vi "EnFlo_Tunnel_Display.vi"(4 "End Time":dbl, 5 "Start Time":dbl, 6 "Channel Values":dbl[](array[numeric]) format="%.3f", 7 "Ch names":string[](array[string])) -> ()   [LabVIEW 2015]
uses:
  Anemometry Sub Vis/Data_plotting_vis/File_Template_Clus.ctl
  Anemometry Sub Vis/Controls/Global_mode.ctl
  Anemometry Sub Vis/Globals/Constants_global.vi
  Anemometry Sub Vis/Data_plotting_vis/Results_plotter_Global.vi
  <vilib>/gmath/NI_Gmath.lvlib
panel:
  out "Averaging time (minutes)":dbl format="%#.1f"
  out "End time":timestamp format="%<%H:%M\n%x>T"
  out "Start time":timestamp format="%<%H:%M\n%x>T"
  out "Top Level":bool
  out "Loop number":i32
  out "Lateral profiles":cluster{"Y Axis Current":dbl[], dbl[]}[](graph)
  out "Setpoints":dbl[](array[numeric])
  in  "Subtract Setpoint?":bool
  out "Vert Disp (mm)  @ 14m":dbl
  out "Inlet St Dev":dbl format="%#.3g"
  out "Inlet mapping":dbl[][](graph)=[[0.00729, 0.18153463174730816, 0.17352738437348433, 1.6752433719500537, 8.231465735195274, 17.570357598383207, 23.099772817121426, 25.58386930448374, 25.31727725753219, 24.28926231541072, 18.717383219374323, 10.355253339797807, 2.7760273383248344, 0.3109897541921306, 0.08276881403435009, 0.06197], [0.04411, 0.1361526368018142, 0.04039202183336771, 1.5611636795339547, 8.176972694107874, 17.32000974741714, 24.257541358764026, 25.949153465972987, 26.01802540761648, 25.060373307424115, 18.284750328365213, 8.689831176707928, 2.642937641487066, 0.43219350072447926, -0.019957690739617468, 0.07351], [0.05478, 0.03446320268089581, 0.2086595806581808, 1.6919212249796047, 6.580368005180591, 14.333585185483123, 21.06810094963999, 23.709254571137723, 24.04768940379576, 21.01660820522005, 13.60443428327954, 6.2766496258038735, 1.7988963349022484, 0.2952877651784204, 0.05436788410934033, 0.1022], [0.04013, 0.06419557464541133, 0.2035068586120256, 1.3118741659450193, 4.7061387064566835, 9.009825946069038, 12.927700276268434, 17.003135081884164, 16.83885730812343, 12.902263313363814, 8.246161922417906, 4.035269404379355, 1.329605659745338, 0.24574055091433544, 0.012829784119986217, 0.08755], [0.04404, 0.022691144295571734, 0.19102098261858932, 0.8525411026079828, 2.2353542219792946, 3.966676465246214, 6.305347763088489, 8.17672908183636, 7.7348668140659, 5.703994479070454, 3.8329088824353237, 1.9256956625267279, 0.6611488869641811, 0.20508248283573002, 0.10119553469307395, 0.08441]]
  out "Upstream Floor":cluster{"Array":dbl[], dbl[]}[](graph)
  in  "Averaging time (mins)":dbl=0.5 format="%.2f"
  in  "History in Minutes":dbl
  out "Strat":cluster{dbl[], dbl[]}[](graph)
  out "Des Air Temp":dbl format="%#.2g"
  out "Heat Extraction kW":dbl format="%#.2g"
  out "Av Pre Inlet Temp":dbl format="%#.2g"
  out "Av Exit  Temp":dbl format="%#.2g"
  out "Exit Dem Temp":dbl format="%#.2g"
  out "Heat Exchanger Valve %":dbl format="%#.1f"
  out "Delta T":dbl format="%#.2g"
  out "Pump Speed %":dbl format="%#.0f"
  out "Meas Delta P":dbl format="%#.2g"
  out "Desired Delta P":dbl format="%#.2f"
  out "Return Pressure":dbl format="%#.2g"
  out "Supply Pressure":dbl format="%#.2g"
  out "Max Motor Temp":dbl format="%#.1g"
  out "% Speed Tweak":dbl format="%#.2g"
  out "Shaft RPM":dbl format="%#.2g"
  out "K Factor":dbl format="%#.2g"
  out "Tunnel Speed  m/s":dbl format="%.3g"
  out "Uni Chilled water Temp":dbl format="%#.2g"
  out "Mixing Valve %":dbl format="%#.1f"
  out "Dem Temp":dbl
  out "Return Temp":dbl format="%#.2g"
  out "Supply Temp":dbl format="%#.2g"
  out "Floor_Cooling:Enable":bool
  out "Chiller_Pump:Enable":bool
  out "Panel Temps":cluster{"Array":dbl[], dbl[]}[](graph)
  in  "Stop Button":bool
  out "Heaters Enabled":bool
  out "Inlet Heaters":cluster{"yi":dbl[], dbl[]}[](graph)
  # "Chiller Pump Information"
  # "Chilled Water"
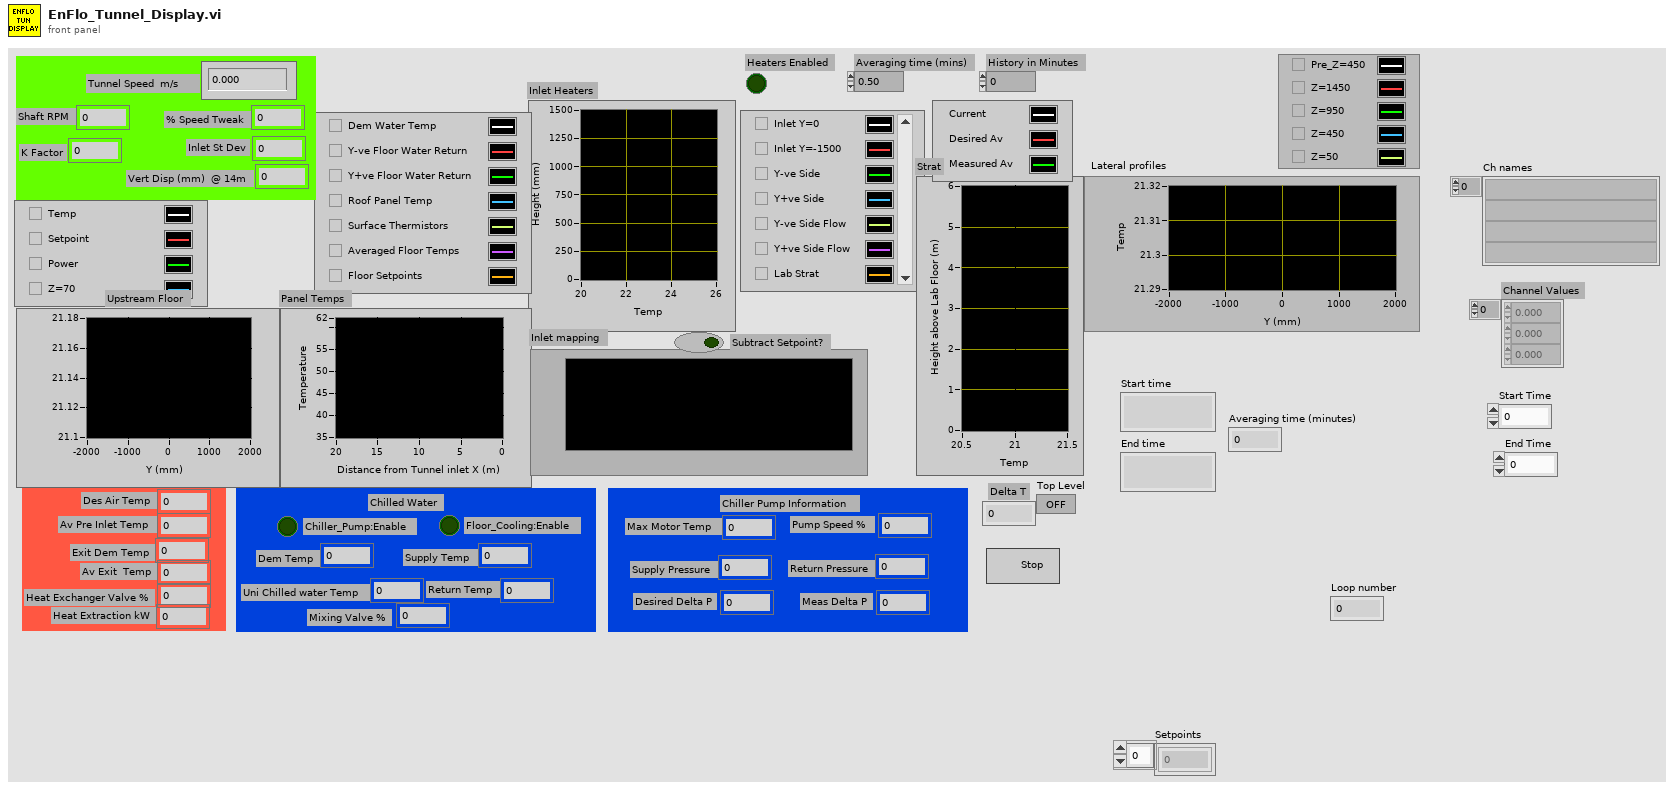
[diagram p1: front panel]
types:
  T1 = typedef "Global_mode.ctl" = enum16{"Read Global", "Load Global From File", "Write Global to File"}
  T2 = typedef "File_Template_Clus.ctl" = cluster{"Template Channel Name":string, "Description":string, "Tolerance":dbl, "Precision":string, "Folder level":string, "Source":string[], "Replace":string[], "Summarise":bool, "Dispose":bool, "Minimum Value":string, "Maths":string, "Omit Rows Containing":string[], "Ignore When":string[]}
  T3 = cluster{"X Max":dbl, "Y Max ":dbl, "X Scale":cluster{"Xo":dbl, "delta X":dbl}, "Y Scale":cluster{"Xo":dbl, "delta X":dbl}, "X Values":dbl[], "Y Values":dbl[], "Z Max":dbl, "Z Min":dbl}
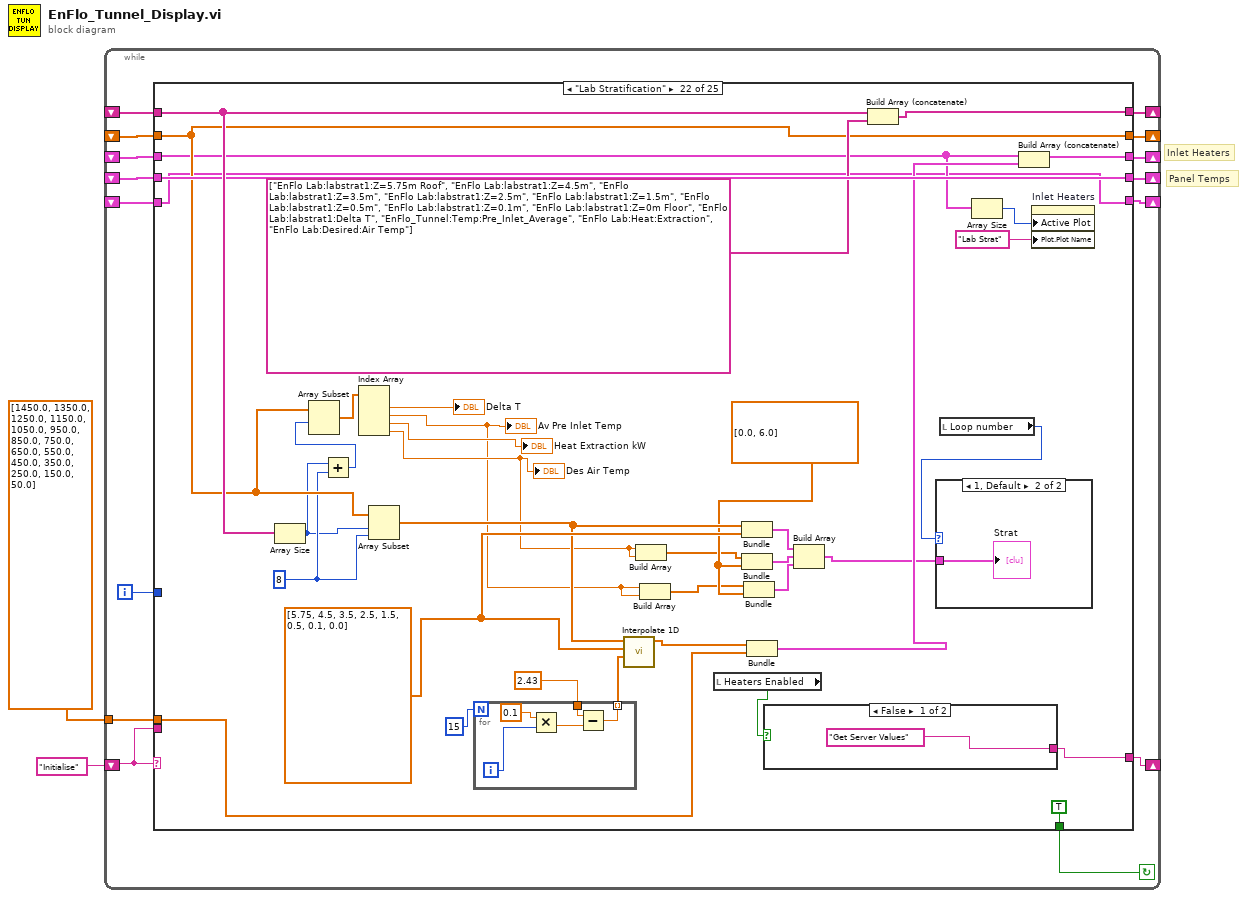
[diagram p0: block diagram]
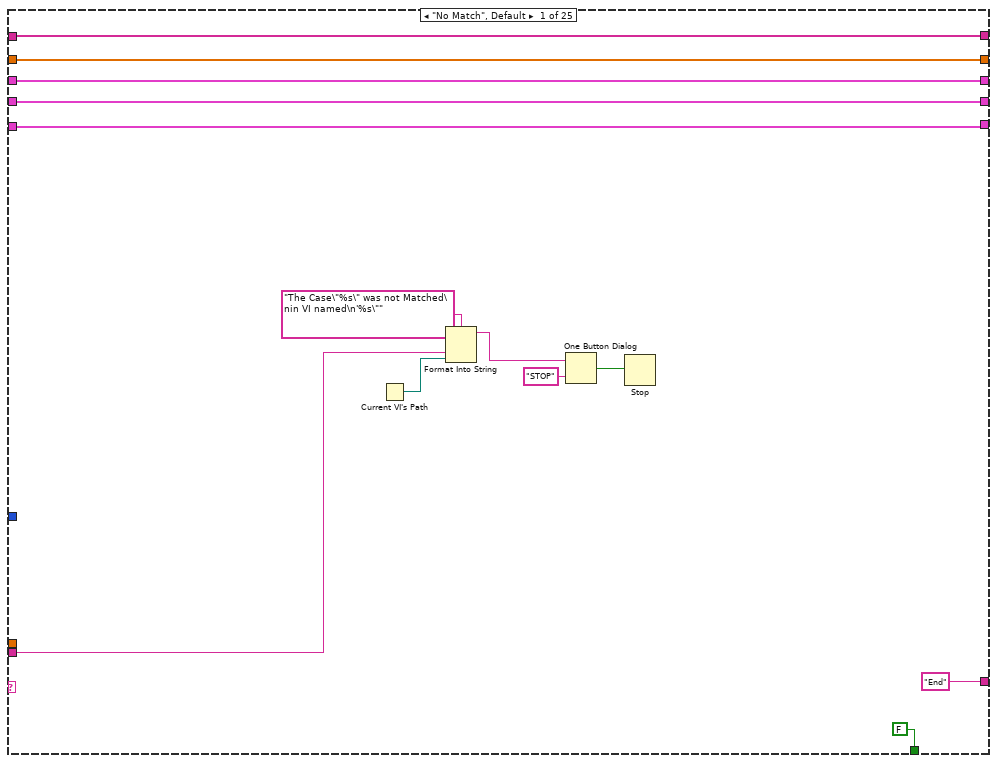
[diagram p2: hidden frame]
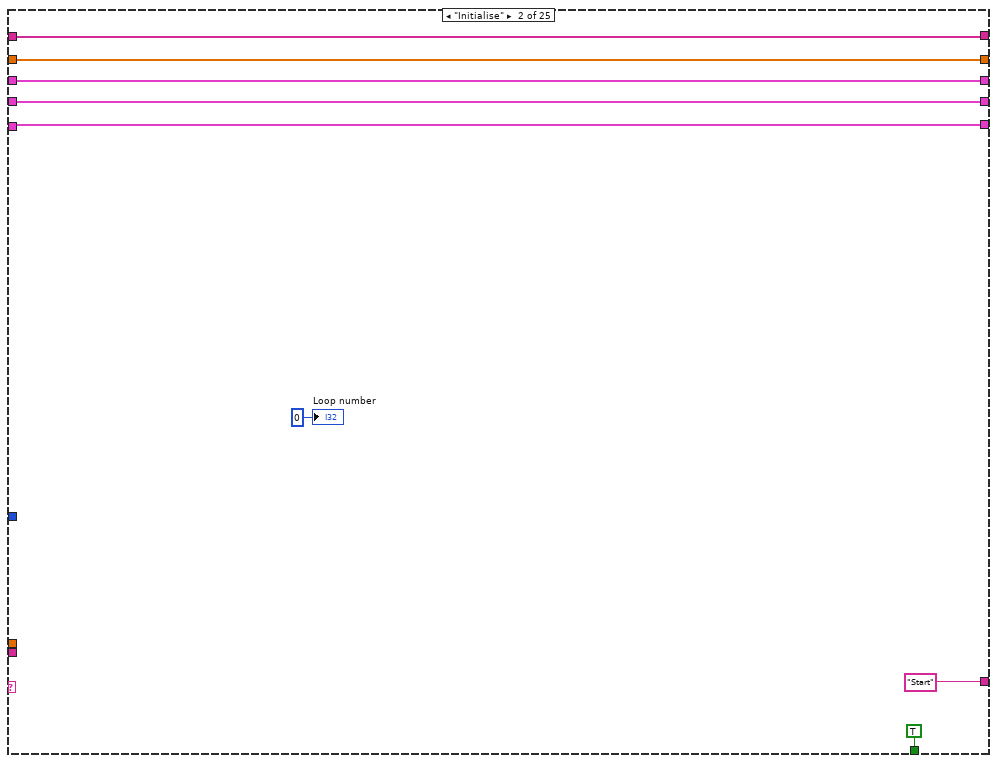
[diagram p3: hidden frame]
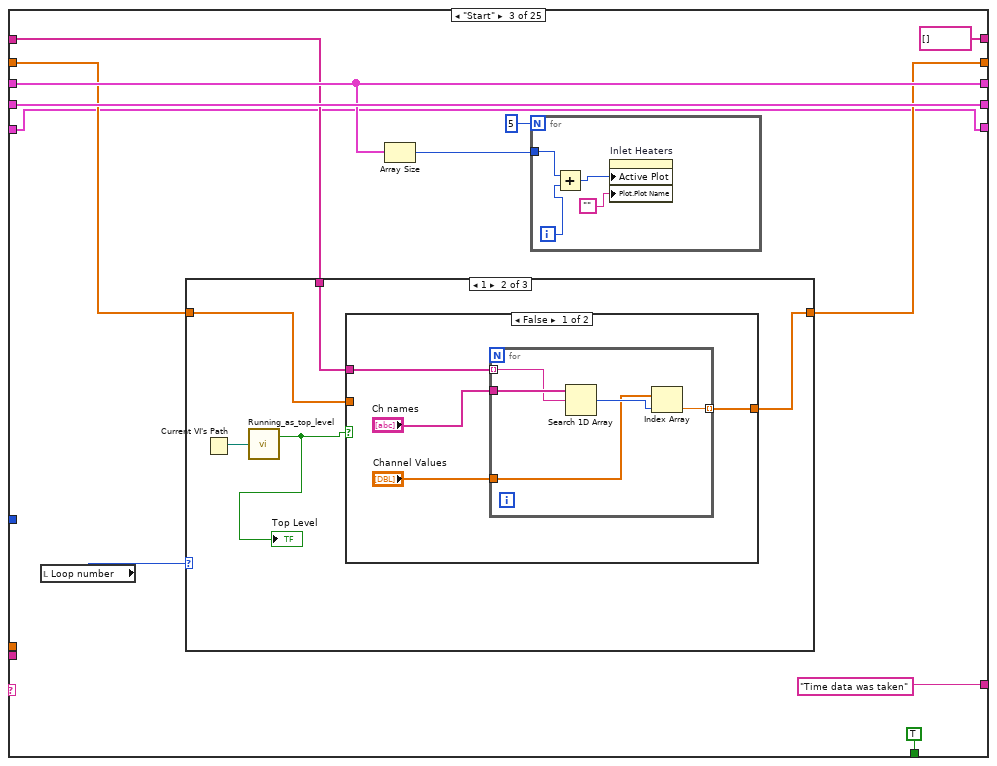
[diagram p4: hidden frame]
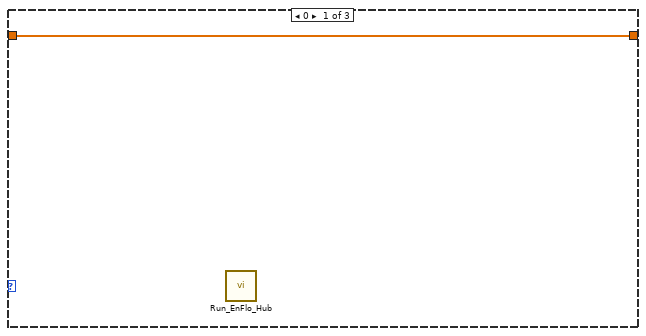
[diagram p5: hidden frame]
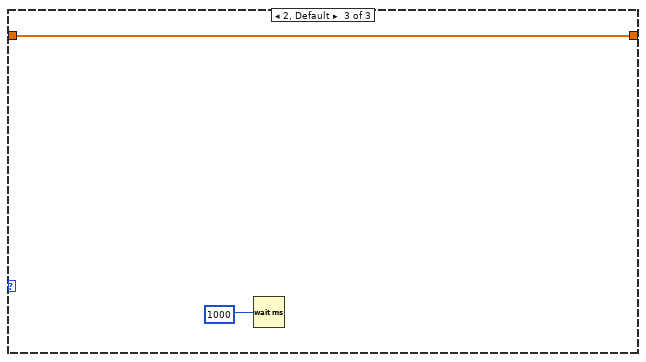
[diagram p7: hidden frame]
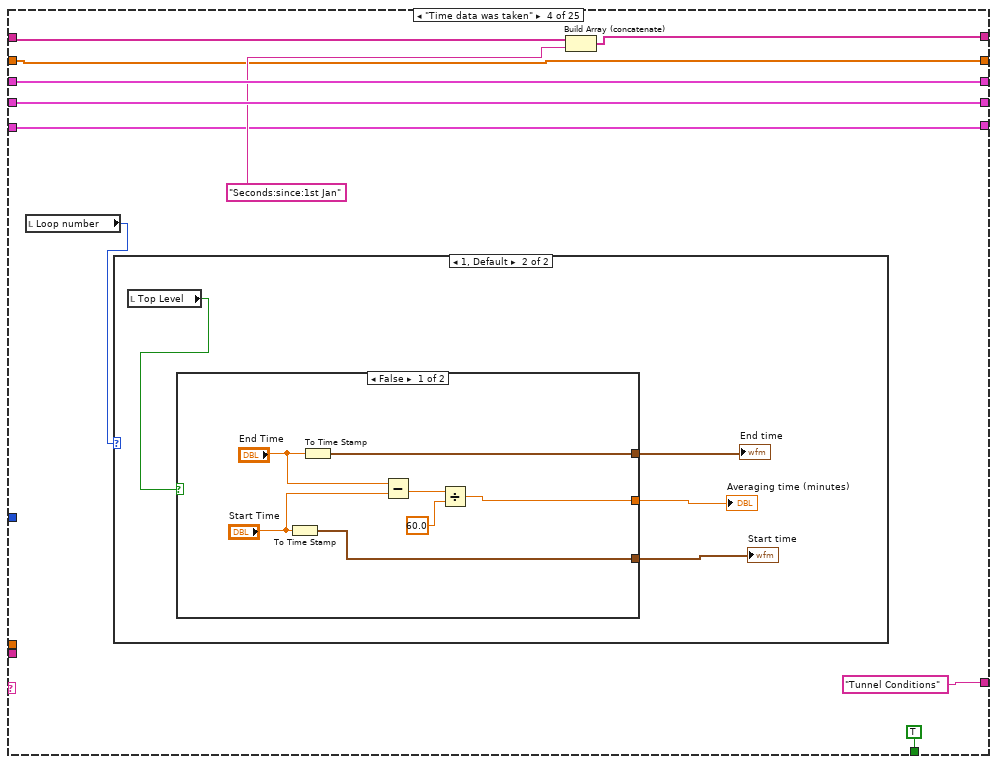
[diagram p8: hidden frame]
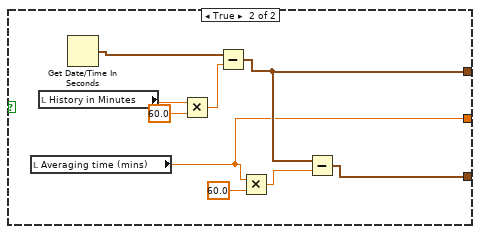
[diagram p10: hidden frame]
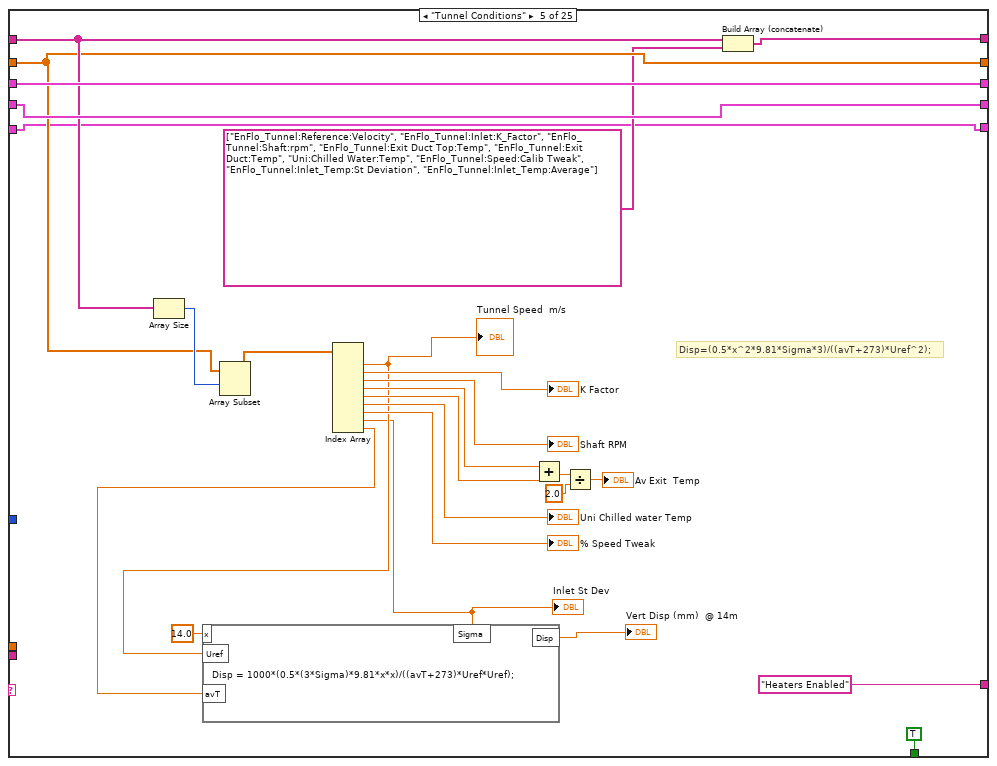
[diagram p11: hidden frame]
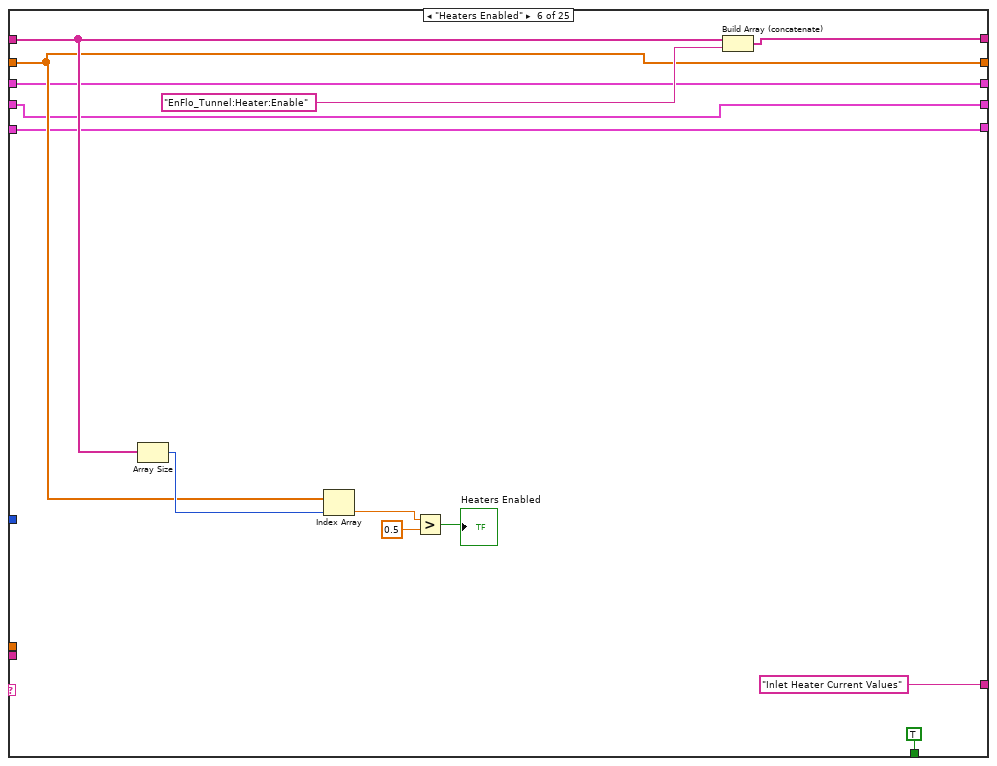
[diagram p12: hidden frame]
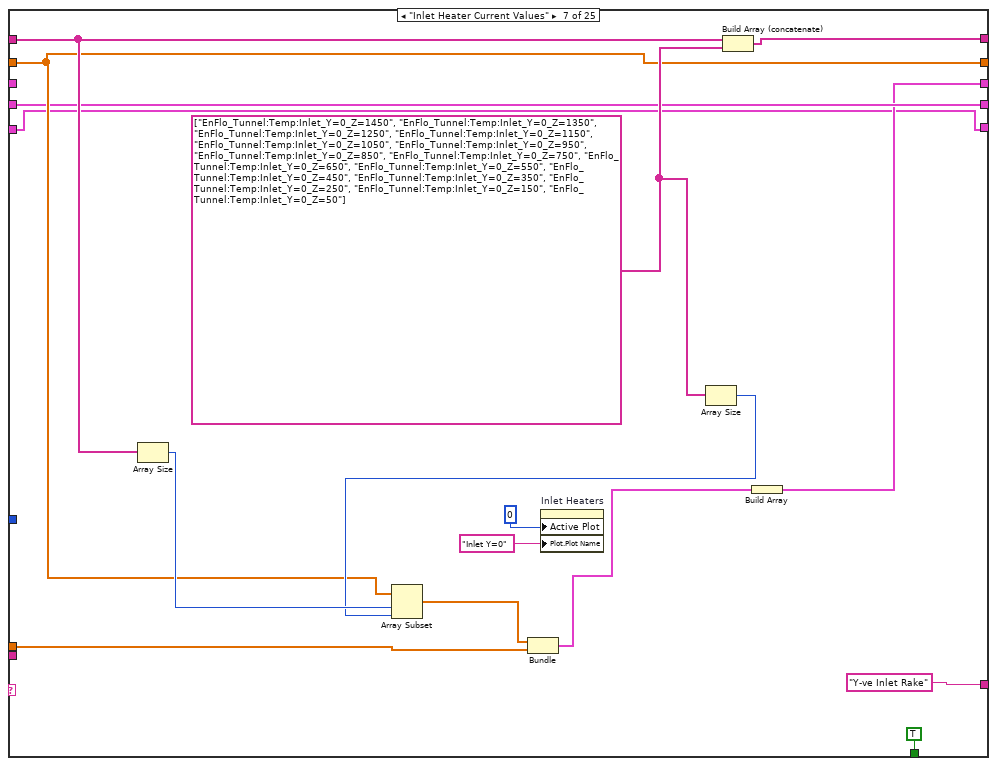
[diagram p13: hidden frame]
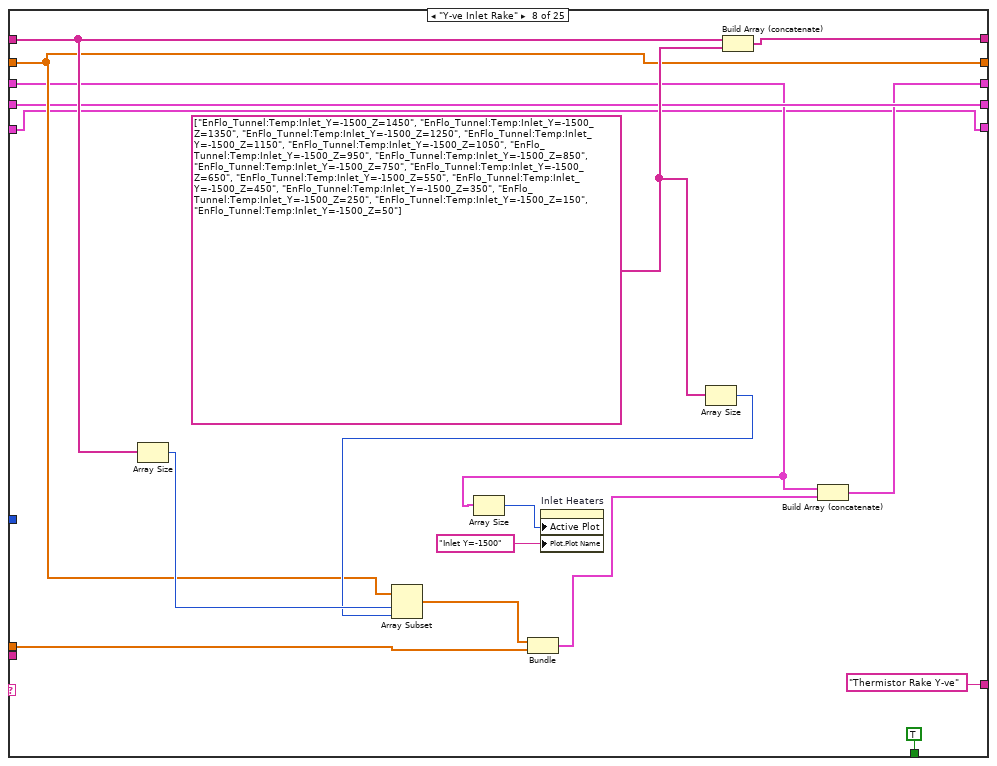
[diagram p14: hidden frame]
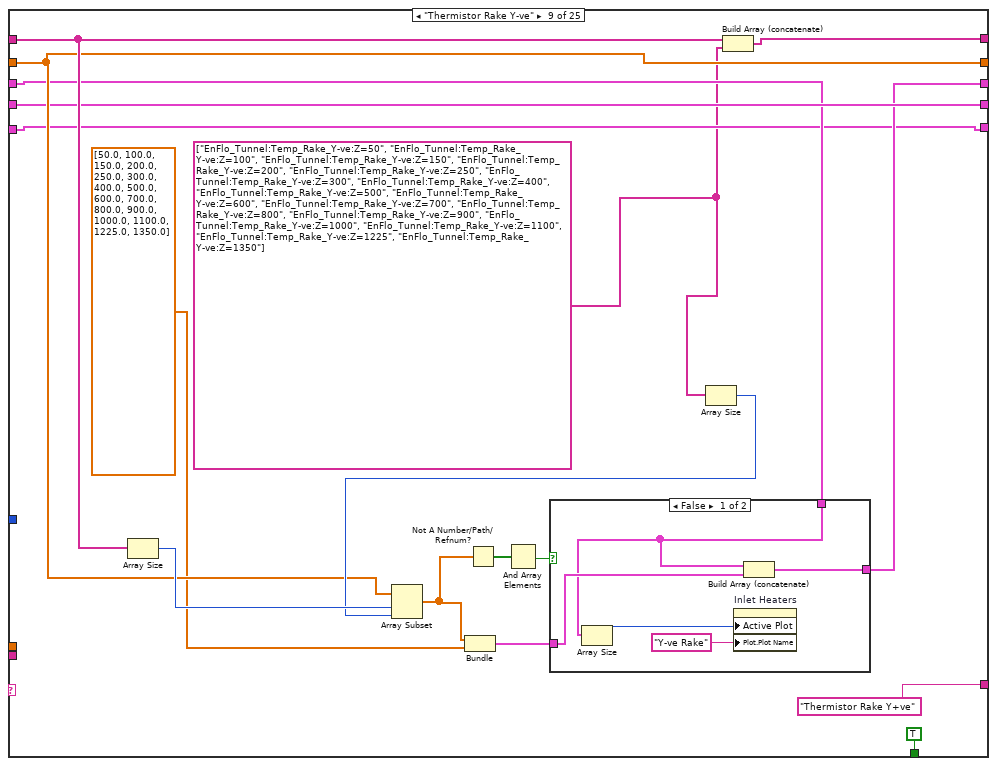
[diagram p15: hidden frame]
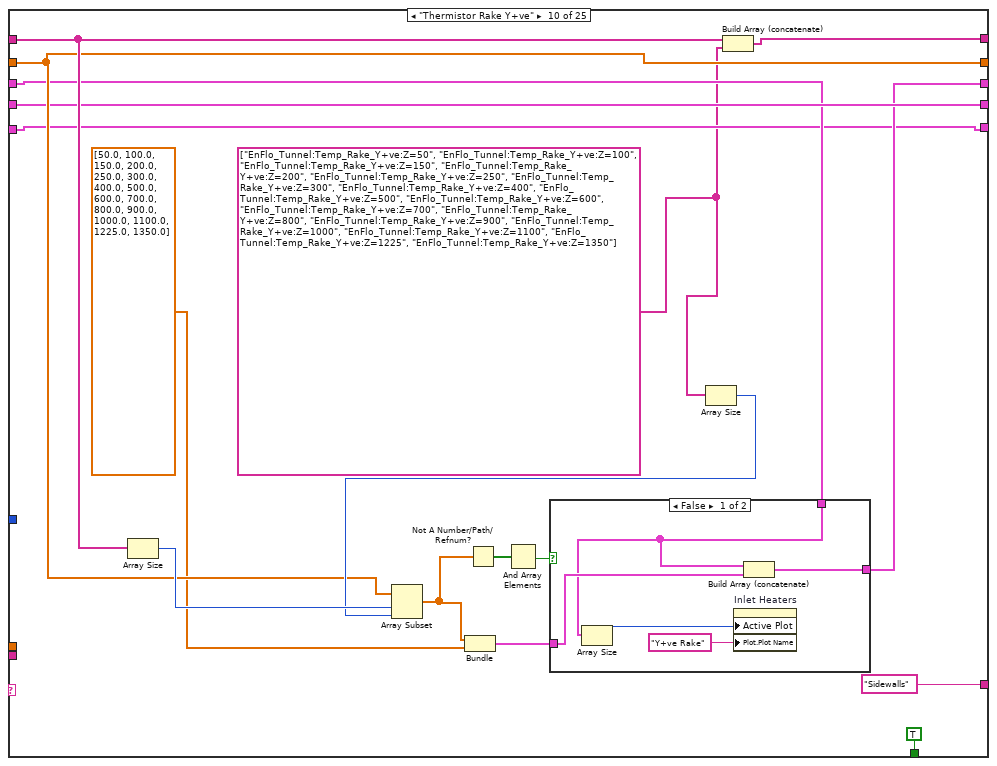
[diagram p17: hidden frame]
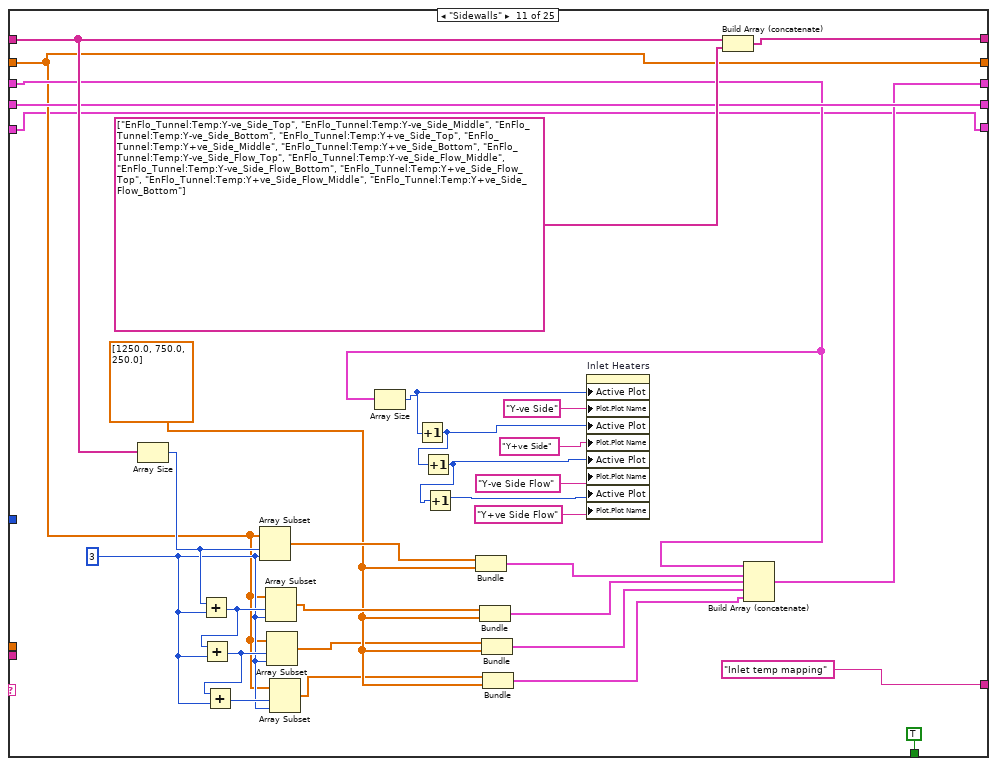
[diagram p19: hidden frame]
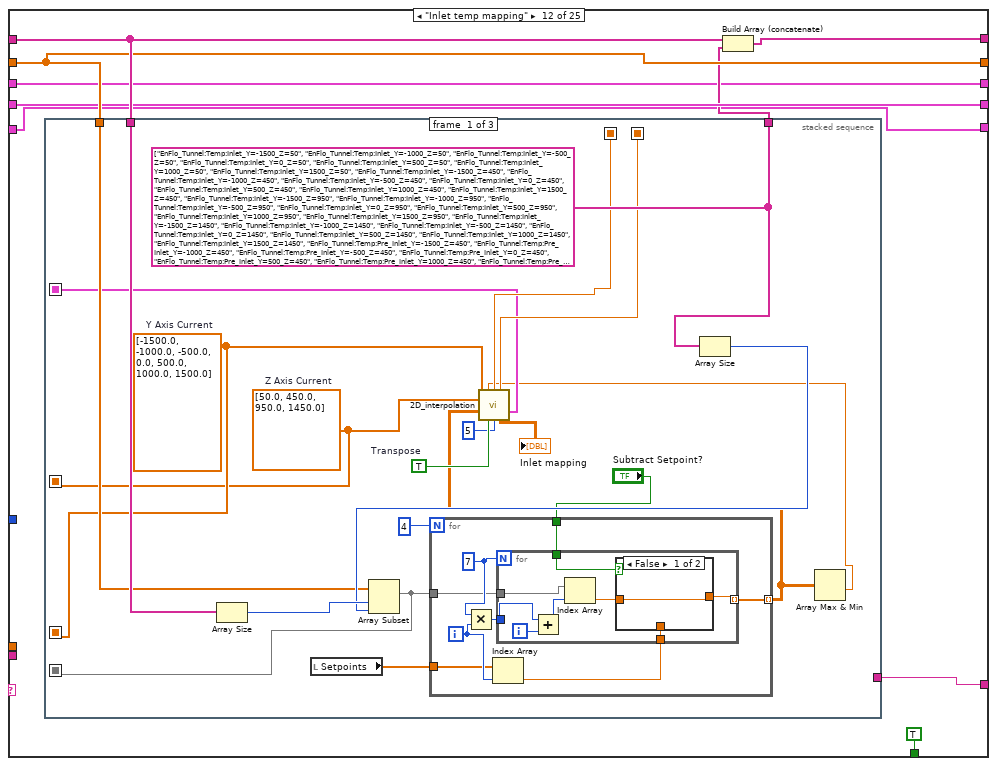
[diagram p20: hidden frame]
diagram:
  # "Panel Temps"
  # "Inlet Heaters"
  n1 = while {
    shift-right: [w15] -> _
    shift-left: "Initialise" -> [w16]
    shift-right: [w14] -> _
    shift-left: _ -> [w13]
    shift-right: [w11] -> _
    shift-left: _ -> [w12]
    shift-right: [w9] -> _
    shift-left: _ -> [w10]
    shift-right: [w8] -> _
    shift-left: _ -> [w7]
    tunnel: dbl[] [1450.0, 1350.0, 1250.0, 1150.0, 1050.0, 950.0, 850.0, 750.0, 650.0, 550.0, 450.0, 350.0, 250.0, 150.0, 50.0] -> [w5]
    shift-right: [w3] -> _
    shift-left: _ -> [w4]
    i -> [w6]
    stop <- w17 continue-if-true
    n2 = case shown="\"Lab Stratification\"" w16 {
      tunnel: [FALSE TRUE ("Top Level") TRUE TRUE ("Top Level") TRUE TRUE TRUE TRUE TRUE TRUE TRUE TRUE TRUE TRUE TRUE TRUE TRUE TRUE TRUE TRUE TRUE TRUE TRUE TRUE w594] -> w17
      tunnel: w16 -> [w24 _ _ _ _ _ _ _ _ _ _ _ _ _ _ _ _ _ _ _ _ _ _ _ _]
      tunnel: ["End" "Start" "Time data was taken" "Tunnel Conditions" "Heaters Enabled" "Inlet Heater Current Values" "Y-ve Inlet Rake" "Thermistor Rake Y-ve" "Thermistor Rake Y+ve" "Sidewalls" "Inlet temp mapping" w253 "EnFlo_Tunnel Chilled Water info" "EnFlo_Tunnel:Floor_Cooling:Enable" "Floor Panels Return Temps" "Roof Panel Values" "Upstream Floor Panel Temps" "Upstream Floor Panel Setpoints" "Upstream Floor Panel Powers" "Upstream Above Floor Panel" "Lab Stratification" w505 "Inlet Heater Power Values" "Get Server Values" "Start"] -> w15
      tunnel: [w22 w34 string[] [] w79 w125 w138 w154 w171 w189 w212 w249 w259 w340 w367 w380 w403 w433 w449 w466 w483 w500 w538 w565 w585 w591] -> w14
      tunnel: w13 -> [w22 w34 w41 w78 w120 w137 w153 w170 w188 w211 w248 w258 w339 w366 w379 w402 w432 w448 w465 w482 w499 w537 w564 w584 w591]
      tunnel: w12 -> [w21 w35 w42 w75 w119 w134 w150 w167 w185 w208 w223 w257 w336 w361 w376 w399 w429 w445 w462 w479 w496 w524 w561 w581 _]
      tunnel: [w21 w35 w43 w75 w119 w134 w150 w167 w185 w208 w223 w257 w336 w361 w376 w399 w429 w445 w462 w479 w496 w524 w561 w581 w593] -> w11
      tunnel: w10 -> [w20 w38 w47 w82 w124 w133 _ w159 w181 w204 w238 w254 w335 w365 w375 w397 w428 w444 w461 w478 w495 w507 w552 w573 w589]
      tunnel: [w20 w38 w47 w82 w124 w133 w143 w162 w182 w205 w244 w254 w335 w365 w375 w397 w428 w444 w461 w478 w495 w528 w559 w577 w589] -> w9
      tunnel: w7 -> [w19 w37 w48 w81 w123 w129 w149 w166 w184 w207 w247 w256 w331 w364 w371 _ w427 w440 w457 w474 w491 w536 w558 w579 w590]
      tunnel: [w19 w37 w48 w81 w123 w129 w149 w166 w184 w207 w247 w256 w331 w364 w371 w384 w426 w440 w457 w474 w491 w536 w558 w579 w590] -> w8
      tunnel: w6 -> [_ _ _ _ _ _ _ _ _ _ _ _ _ _ _ _ _ _ _ _ _ _ _ _ _]
      tunnel: w5 -> [_ _ _ _ _ _ w147 w164 _ _ _ _ _ _ _ _ _ _ _ _ _ w510 w553 w578 _]
      tunnel: w4 -> [w18 w31 w39 w73 w103 w128 w141 w157 w176 w199 w220 w252 w329 w342 w369 w382 w421 _ w454 w471 w488 w503 w548 w570 w587]
      tunnel: [w18 w31 w39 w73 w103 w128 w141 w157 w176 w199 w220 w252 w329 w342 w369 w382 w421 w438 w455 w472 w489 w503 w548 w570 w587] -> w3
      frame "No Match", Default {
        n3 = Current VI's Path() -> (path=w29:path)
        n4 = Format Into String(format string="The Case\"%s\" was not Matched\nin VI named\n'%s\"" ("Format String"), w24, w29) -> (resulting string=w26:string)  [unwired: 2 in, 1 out]
        n5 = One Button Dialog(message=w26, button name ("OK")="STOP") -> (true=w28:bool)
        n6 = Stop(stop? (T)=w28) -> ()
      }
      frame "Initialise" {
        "Loop number" <- 0 ("Loop number")
      }
      frame "Start" {
        n7 = local read "Loop number"() -> (w44:i32)
        n8 = case shown="1" w44 {
          tunnel: [w55 w59 w71] -> w43
          tunnel: w42 -> [w55 w57 w71]
          tunnel: w41 -> [_ w60 _]
          frame 0 {
            n9 = call "Run_EnFlo_Hub.vi"() -> ()  [unwired: 8 in]
          }
          frame 1 {
            n10 = Current VI's Path() -> (path=w58:path)
            n11 = call "Running_as_top_level.vi"("Vi path name"=w58) -> ("Top Level"=w56:bool)  [unwired: 1 out]
            "Top Level" <- w56
            n12 = case shown="False" w56 {
              tunnel: w60 -> [w63 _]
              tunnel: [w61 w70] -> w59
              tunnel: w57 -> [_ w70]
              frame False {
                n13 = for {
                  tunnel: "Ch names" -> [w69]
                  tunnel: w63 -> [w68] mode=indexing
                  tunnel: "Channel Values" -> [w66]
                  tunnel: [w65] -> w61 mode=indexing
                  n14 = Search 1D Array(1D array=w69, element=w68) -> (index of element=w67:i32)  [unwired: 1 in]
                  n15 = Index Array(array=w66, index=w67) -> (element=w65:dbl)
                }
              }
              frame True {
              }
            }
          }
          frame 2, Default {
            n16 = Wait (ms)(milliseconds to wait=u32 1000 ("millisecond timer value")) -> ()  [unwired: 1 out]
          }
        }
        n17 = Array Size(array=w47) -> (size(s)=w45:i32)
        n18 = for {
          N: 5 -> [_]
          tunnel: w45 -> [w54]
          i -> [w53]
          n19 = Add(x=w54, y=w53) -> (x+y=w52:i32)
          n20 = property on="Inlet Heaters" class="XYGraph (strict)"("Active Plot"=w52, "Plot.Plot Name"="") -> ()  [unwired: 2 in, 2 out]
        }
      }
      frame "Time data was taken" {
        n21 = local read "Loop number"() -> (w74:i32)
        n22 = case shown="1, Default" w74 {
          frame 0 {
          }
          frame 1, Default {
            n23 = local read "Top Level"() -> (w84:bool)
            n24 = case shown="False" w84 {
              tunnel: [w93 w100] -> w86
              tunnel: [w92 w101] -> w85
              tunnel: [w87 w94] -> w83
              frame False {
                n25 = To Time Stamp(1:"Start Time") -> (0:w93:timestamp)
                n26 = To Time Stamp(1:"End Time") -> (0:w92:timestamp)
                n27 = Subtract(x="End Time", y="Start Time") -> (x-y=w89:dbl)
                n28 = Divide(x=w89, y=60.0) -> (x/y=w87:dbl)
              }
              frame True {
                n29 = local read "Averaging time (mins)"() -> (w94:dbl)
                n30 = local read "History in Minutes"() -> (w99:dbl)
                n31 = Get Date/Time In Seconds() -> (seconds since 1Jan1904=w102:timestamp)
                n32 = Multiply(x=w99, y=60.0) -> (x*y=w97:dbl)
                n33 = Subtract(x=w102, y=w97) -> (x-y=w101:timestamp)
                n34 = Multiply(x=w94, y=60.0) -> (x*y=w95:dbl)
                n35 = Subtract(x=w101, y=w95) -> (x-y=w100:timestamp)
              }
            }
            "Start time" <- w86
            "End time" <- w85
            "Averaging time (minutes)" <- w83
          }
        }
        n36 = Build Array (concatenate)(w78, "Seconds:since:1st Jan") -> (w79:string[])
      }
      frame "Tunnel Conditions" {
        # "Disp=(0.5*x^2*9.81*Sigma*3)/((avT+273)*Uref^2);"
        n37 = Array Size(array=w120) -> (size(s)=w122:i32)
        n38 = Array Subset(array=w119, index=w122) -> (w121:dbl[])  [unwired: 1 in]
        n39 = Index Array(array=w121) -> (element #1=w107:dbl, element #2=→"K Factor":dbl, element #3=→"Shaft RPM":dbl, element #4=w112:dbl, element #5=w111:dbl, element #6=→"Uni Chilled water Temp":dbl, element #7=→"% Speed Tweak":dbl, element #8=w105:dbl, element #9=w104:dbl)  [unwired: 9 in]
        "Tunnel Speed  m/s" <- w107
        "Inlet St Dev" <- w105
        n40 = formula code="Disp = 1000*(0.5*(3*Sigma)*9.81*x*x)/((avT+273)*Uref*Uref);"("x"=14.0 ("input variable"), "Uref"=w107, "Sigma"=w105, "avT"=w104) -> ("Disp"=→"Vert Disp (mm)  @ 14m":dbl)
        n41 = Add(x=w112, y=w111) -> (x+y=w116:dbl)
        n42 = Divide(x=w116, y=2.0) -> (x/y=→"Av Exit  Temp":dbl)
        n43 = Build Array (concatenate)(w120, string[] ["EnFlo_Tunnel:Reference:Velocity", "EnFlo_Tunnel:Inlet:K_Factor", "EnFlo_Tunnel:Shaft:rpm", "EnFlo_Tunnel:Exit Duct Top:Temp", "EnFlo_Tunnel:Exit Duct:Temp", "Uni:Chilled Water:Temp", "EnFlo_Tunnel:Speed:Calib Tweak", "EnFlo_Tunnel:Inlet_Temp:St Deviation", "EnFlo_Tunnel:Inlet_Temp:Average"] ("subarray")) -> (w125:string[])
      }
      frame "Heaters Enabled" {
        n44 = Array Size(array=w137) -> (size(s)=w135:i32)
        n45 = Index Array(array=w134, index=w135) -> (element=w132:dbl)
        n46 = Greater?(x=w132, y=0.5) -> (0:→"Heaters Enabled":bool)
        n47 = Build Array (concatenate)(w137, "EnFlo_Tunnel:Heater:Enable" ("Ch Name")) -> (w138:string[])
      }
      frame "Inlet Heater Current Values" {
        w155 = string[] ["EnFlo_Tunnel:Temp:Inlet_Y=0_Z=1450", "EnFlo_Tunnel:Temp:Inlet_Y=0_Z=1350", "EnFlo_Tunnel:Temp:Inlet_Y=0_Z=1250", "EnFlo_Tunnel:Temp:Inlet_Y=0_Z=1150", "EnFlo_Tunnel:Temp:Inlet_Y=0_Z=1050", "EnFlo_Tunnel:Temp:Inlet_Y=0_Z=950", "EnFlo_Tunnel:Temp:Inlet_Y=0_Z=850", "EnFlo_Tunnel:Temp:Inlet_Y=0_Z=750", "EnFlo_Tunnel:Temp:Inlet_Y=0_Z=650", "EnFlo_Tunnel:Temp:Inlet_Y=0_Z=550", "EnFlo_Tunnel:Temp:Inlet_Y=0_Z=450", "EnFlo_Tunnel:Temp:Inlet_Y=0_Z=350", "EnFlo_Tunnel:Temp:Inlet_Y=0_Z=250", "EnFlo_Tunnel:Temp:Inlet_Y=0_Z=150", "EnFlo_Tunnel:Temp:Inlet_Y=0_Z=50"] ("subarray")
        n48 = Array Size(array=w153) -> (size(s)=w152:i32)
        n49 = property on="Inlet Heaters" class="XYGraph (strict)"("Active Plot"=u32 0, "Plot.Plot Name"="Inlet Y=0") -> ()  [unwired: 2 in, 2 out]
        n50 = Array Size(array=w155) -> (size(s)=w151:i32)
        n51 = Array Subset(array=w150, index=w152, length=w151) -> (w148:dbl[])
        n52 = Bundle(w148, w147) -> (w144:cluster{dbl[], dbl[]})  [unwired: 1 in]
        n53 = Build Array (concatenate)(w153, w155) -> (w154:string[])
        n54 = Build Array(w144) -> (w143:cluster{dbl[], dbl[]}[])
      }
      frame "Y-ve Inlet Rake" {
        w172 = string[] ["EnFlo_Tunnel:Temp:Inlet_Y=-1500_Z=1450", "EnFlo_Tunnel:Temp:Inlet_Y=-1500_Z=1350", "EnFlo_Tunnel:Temp:Inlet_Y=-1500_Z=1250", "EnFlo_Tunnel:Temp:Inlet_Y=-1500_Z=1150", "EnFlo_Tunnel:Temp:Inlet_Y=-1500_Z=1050", "EnFlo_Tunnel:Temp:Inlet_Y=-1500_Z=950", "EnFlo_Tunnel:Temp:Inlet_Y=-1500_Z=850", "EnFlo_Tunnel:Temp:Inlet_Y=-1500_Z=750", "EnFlo_Tunnel:Temp:Inlet_Y=-1500_Z=650", "EnFlo_Tunnel:Temp:Inlet_Y=-1500_Z=550", "EnFlo_Tunnel:Temp:Inlet_Y=-1500_Z=450", "EnFlo_Tunnel:Temp:Inlet_Y=-1500_Z=350", "EnFlo_Tunnel:Temp:Inlet_Y=-1500_Z=250", "EnFlo_Tunnel:Temp:Inlet_Y=-1500_Z=150", "EnFlo_Tunnel:Temp:Inlet_Y=-1500_Z=50"] ("subarray")
        n55 = Array Size(array=w170) -> (size(s)=w169:i32)
        n56 = Array Size(array=w159) -> (size(s)=w158:i32)
        n57 = property on="Inlet Heaters" class="XYGraph (strict)"("Active Plot"=w158, "Plot.Plot Name"="Inlet Y=-1500") -> ()  [unwired: 2 in, 2 out]
        n58 = Array Size(array=w172) -> (size(s)=w168:i32)
        n59 = Array Subset(array=w167, index=w169, length=w168) -> (w165:dbl[])
        n60 = Bundle(w165, w164) -> (w160:cluster{dbl[], dbl[]})  [unwired: 1 in]
        n61 = Build Array (concatenate)(w170, w172) -> (w171:string[])
        n62 = Build Array (concatenate)(w159, w160) -> (w162:cluster{"yi":dbl[], dbl[]}[])
      }
      frame "Thermistor Rake Y-ve" {
        w175 = string[] ["EnFlo_Tunnel:Temp_Rake_Y-ve:Z=50", "EnFlo_Tunnel:Temp_Rake_Y-ve:Z=100", "EnFlo_Tunnel:Temp_Rake_Y-ve:Z=150", "EnFlo_Tunnel:Temp_Rake_Y-ve:Z=200", "EnFlo_Tunnel:Temp_Rake_Y-ve:Z=250", "EnFlo_Tunnel:Temp_Rake_Y-ve:Z=300", "EnFlo_Tunnel:Temp_Rake_Y-ve:Z=400", "EnFlo_Tunnel:Temp_Rake_Y-ve:Z=500", "EnFlo_Tunnel:Temp_Rake_Y-ve:Z=600", "EnFlo_Tunnel:Temp_Rake_Y-ve:Z=700", "EnFlo_Tunnel:Temp_Rake_Y-ve:Z=800", "EnFlo_Tunnel:Temp_Rake_Y-ve:Z=900", "EnFlo_Tunnel:Temp_Rake_Y-ve:Z=1000", "EnFlo_Tunnel:Temp_Rake_Y-ve:Z=1100", "EnFlo_Tunnel:Temp_Rake_Y-ve:Z=1225", "EnFlo_Tunnel:Temp_Rake_Y-ve:Z=1350"] ("Sub set")
        n63 = Array Size(array=w188) -> (size(s)=w187:i32)
        n64 = Array Size(array=w175) -> (size(s)=w186:i32)
        n65 = Array Subset(array=w185, index=w187, length=w186) -> (w180:dbl[])
        n66 = Bundle(w180, dbl[] [50.0, 100.0, 150.0, 200.0, 250.0, 300.0, 400.0, 500.0, 600.0, 700.0, 800.0, 900.0, 1000.0, 1100.0, 1225.0, 1350.0]) -> (w177:cluster{dbl[], dbl[]})  [unwired: 1 in]
        n67 = Not A Number/Path/Refnum?(number/path/refnum=w180) -> (NaN/Path/Refnum?=w179:bool[])
        n68 = And Array Elements(Boolean array=w179) -> (logical AND=w178:bool)
        n69 = case shown="False" w178 {
          tunnel: [w195 w196] -> w182
          tunnel: w181 -> [w191 w196]
          tunnel: w177 -> [w194 _]
          frame False {
            n70 = Array Size(array=w191) -> (size(s)=w192:i32)
            n71 = property on="Inlet Heaters" class="XYGraph (strict)"("Active Plot"=w192, "Plot.Plot Name"="Y-ve Rake") -> ()  [unwired: 2 in, 2 out]
            n72 = Build Array (concatenate)(w191, w194) -> (w195:cluster{"yi":dbl[], dbl[]}[])
          }
          frame True {
          }
        }
        n73 = Build Array (concatenate)(w188, w175) -> (w189:string[])
      }
      frame "Thermistor Rake Y+ve" {
        w197 = string[] ["EnFlo_Tunnel:Temp_Rake_Y+ve:Z=50", "EnFlo_Tunnel:Temp_Rake_Y+ve:Z=100", "EnFlo_Tunnel:Temp_Rake_Y+ve:Z=150", "EnFlo_Tunnel:Temp_Rake_Y+ve:Z=200", "EnFlo_Tunnel:Temp_Rake_Y+ve:Z=250", "EnFlo_Tunnel:Temp_Rake_Y+ve:Z=300", "EnFlo_Tunnel:Temp_Rake_Y+ve:Z=400", "EnFlo_Tunnel:Temp_Rake_Y+ve:Z=500", "EnFlo_Tunnel:Temp_Rake_Y+ve:Z=600", "EnFlo_Tunnel:Temp_Rake_Y+ve:Z=700", "EnFlo_Tunnel:Temp_Rake_Y+ve:Z=800", "EnFlo_Tunnel:Temp_Rake_Y+ve:Z=900", "EnFlo_Tunnel:Temp_Rake_Y+ve:Z=1000", "EnFlo_Tunnel:Temp_Rake_Y+ve:Z=1100", "EnFlo_Tunnel:Temp_Rake_Y+ve:Z=1225", "EnFlo_Tunnel:Temp_Rake_Y+ve:Z=1350"] ("Sub set")
        n74 = Array Size(array=w211) -> (size(s)=w210:i32)
        n75 = Array Size(array=w197) -> (size(s)=w209:i32)
        n76 = Array Subset(array=w208, index=w210, length=w209) -> (w203:dbl[])
        n77 = Bundle(w203, dbl[] [50.0, 100.0, 150.0, 200.0, 250.0, 300.0, 400.0, 500.0, 600.0, 700.0, 800.0, 900.0, 1000.0, 1100.0, 1225.0, 1350.0]) -> (w200:cluster{dbl[], dbl[]})  [unwired: 1 in]
        n78 = Not A Number/Path/Refnum?(number/path/refnum=w203) -> (NaN/Path/Refnum?=w202:bool[])
        n79 = And Array Elements(Boolean array=w202) -> (logical AND=w201:bool)
        n80 = case shown="False" w201 {
          tunnel: [w218 w219] -> w205
          tunnel: w204 -> [w214 w219]
          tunnel: w200 -> [w217 _]
          frame False {
            n81 = Array Size(array=w214) -> (size(s)=w215:i32)
            n82 = property on="Inlet Heaters" class="XYGraph (strict)"("Active Plot"=w215, "Plot.Plot Name"="Y+ve Rake") -> ()  [unwired: 2 in, 2 out]
            n83 = Build Array (concatenate)(w214, w217) -> (w218:cluster{"yi":dbl[], dbl[]}[])
          }
          frame True {
          }
        }
        n84 = Build Array (concatenate)(w211, w197) -> (w212:string[])
      }
      frame "Sidewalls" {
        w226 = dbl[] [1250.0, 750.0, 250.0]
        w227 = 3 ("length")
        n85 = Array Size(array=w248) -> (size(s)=w243:i32)
        n86 = Add(x=w243, y=w227) -> (x+y=w229:i32)
        n87 = Add(x=w229, y=w227) -> (x+y=w228:i32)
        n88 = Add(x=w228, y=w227) -> (x+y=w230:i32)
        n89 = Array Subset(array=w223, index=w243, length=w227) -> (w242:dbl[])
        n90 = Array Subset(array=w223, index=w229, length=w227) -> (w241:dbl[])
        n91 = Array Subset(array=w223, index=w228, length=w227) -> (w225:dbl[])
        n92 = Array Subset(array=w223, index=w230, length=w227) -> (w224:dbl[])
        n93 = Array Size(array=w238) -> (size(s)=w236:i32)
        n94 = Increment(x=w236) -> (x+1=w233:i32)
        n95 = Increment(x=w233) -> (x+1=w231:i32)
        n96 = Increment(x=w231) -> (x+1=w232:i32)
        n97 = Bundle(w242, w226) -> (w245:cluster{dbl[], dbl[]})  [unwired: 1 in]
        n98 = Bundle(w241, w226) -> (w240:cluster{dbl[], dbl[]})  [unwired: 1 in]
        n99 = Bundle(w225, w226) -> (w222:cluster{dbl[], dbl[]})  [unwired: 1 in]
        n100 = Bundle(w224, w226) -> (w221:cluster{dbl[], dbl[]})  [unwired: 1 in]
        n101 = property on="Inlet Heaters" class="XYGraph (strict)"("Active Plot"=w236, "Plot.Plot Name"="Y-ve Side", "Active Plot"=w233, "Plot.Plot Name"="Y+ve Side", "Active Plot"=w231, "Plot.Plot Name"="Y-ve Side Flow", "Active Plot"=w232, "Plot.Plot Name"="Y+ve Side Flow") -> ()  [unwired: 2 in, 2 out]
        n102 = Build Array (concatenate)(w248, string[] ["EnFlo_Tunnel:Temp:Y-ve_Side_Top", "EnFlo_Tunnel:Temp:Y-ve_Side_Middle", "EnFlo_Tunnel:Temp:Y-ve_Side_Bottom", "EnFlo_Tunnel:Temp:Y+ve_Side_Top", "EnFlo_Tunnel:Temp:Y+ve_Side_Middle", "EnFlo_Tunnel:Temp:Y+ve_Side_Bottom", "EnFlo_Tunnel:Temp:Y-ve_Side_Flow_Top", "EnFlo_Tunnel:Temp:Y-ve_Side_Flow_Middle", "EnFlo_Tunnel:Temp:Y-ve_Side_Flow_Bottom", "EnFlo_Tunnel:Temp:Y+ve_Side_Flow_Top", "EnFlo_Tunnel:Temp:Y+ve_Side_Flow_Middle", "EnFlo_Tunnel:Temp:Y+ve_Side_Flow_Bottom"] ("subarray")) -> (w249:string[])
        n103 = Build Array (concatenate)(w238, w245, w240, w222, w221) -> (w244:cluster{"yi":dbl[], dbl[]}[])
      }
      frame "Inlet temp mapping" {
        n104 = stacked-sequence {
          seq-local: [w271 _ _] -> [_ w308 _]
          seq-local: [w270 _ _] -> [_ w309 _]
          seq-local: [w269 _ _] -> [_ w304 _]
          seq-local: [w263 _ _] -> [_ _ w319]
          seq-local: [w262 _ _] -> [_ _ w320]
          seq-local: [w261 _ _] -> [_ _ _]
          tunnel: w258 -> [w279 _ _]
          tunnel: w257 -> [w276 _ _]
          tunnel: [w275 _ _] -> w255
          tunnel: [_ "EnFlo_Tunnel:Chiller_Pump:Enable" _] -> w253
          frame #0 {
            w273 = TRUE  # Transpose
            w261 = dbl[] [50.0, 450.0, 950.0, 1450.0]  # Z Axis Current
            w262 = dbl[] [-1500.0, -1000.0, -500.0, 0.0, 500.0, 1000.0, 1500.0]  # Y Axis Current
            w275 = string[] ["EnFlo_Tunnel:Temp:Inlet_Y=-1500_Z=50", "EnFlo_Tunnel:Temp:Inlet_Y=-1000_Z=50", "EnFlo_Tunnel:Temp:Inlet_Y=-500_Z=50", "EnFlo_Tunnel:Temp:Inlet_Y=0_Z=50", "EnFlo_Tunnel:Temp:Inlet_Y=500_Z=50", "EnFlo_Tunnel:Temp:Inlet_Y=1000_Z=50", "EnFlo_Tunnel:Temp:Inlet_Y=1500_Z=50", "EnFlo_Tunnel:Temp:Inlet_Y=-1500_Z=450", "EnFlo_Tunnel:Temp:Inlet_Y=-1000_Z=450", "EnFlo_Tunnel:Temp:Inlet_Y=-500_Z=450", "EnFlo_Tunnel:Temp:Inlet_Y=0_Z=450", "EnFlo_Tunnel:Temp:Inlet_Y=500_Z=450", "EnFlo_Tunnel:Temp:Inlet_Y=1000_Z=450", "EnFlo_Tunnel:Temp:Inlet_Y=1500_Z=450", "EnFlo_Tunnel:Temp:Inlet_Y=-1500_Z=950", "EnFlo_Tunnel:Temp:Inlet_Y=-1000_Z=950", "EnFlo_Tunnel:Temp:Inlet_Y=-500_Z=950", "EnFlo_Tunnel:Temp:Inlet_Y=0_Z=950", "EnFlo_Tunnel:Temp:Inlet_Y=500_Z=950", "EnFlo_Tunnel:Temp:Inlet_Y=1000_Z=950", "EnFlo_Tunnel:Temp:Inlet_Y=1500_Z=950", "EnFlo_Tunnel:Temp:Inlet_Y=-1500_Z=1450", "EnFlo_Tunnel:Temp:Inlet_Y=-1000_Z=1450", "EnFlo_Tunnel:Temp:Inlet_Y=-500_Z=1450", "EnFlo_Tunnel:Temp:Inlet_Y=0_Z=1450", "EnFlo_Tunnel:Temp:Inlet_Y=500_Z=1450", "EnFlo_Tunnel:Temp:Inlet_Y=1000_Z=1450", "EnFlo_Tunnel:Temp:Inlet_Y=1500_Z=1450", "EnFlo_Tunnel:Temp:Pre_Inlet_Y=-1500_Z=450", "EnFlo_Tunnel:Temp:Pre_Inlet_Y=-1000_Z=450", "EnFlo_Tunnel:Temp:Pre_Inlet_Y=-500_Z=450", "EnFlo_Tunnel:Temp:Pre_Inlet_Y=0_Z=450", "EnFlo_Tunnel:Temp:Pre_Inlet_Y=500_Z=450", "EnFlo_Tunnel:Temp:Pre_Inlet_Y=1000_Z=450", "EnFlo_Tunnel:Temp:Pre_Inlet_Y=1500_Z=450"] ("subarray")
            n105 = Array Size(array=w279) -> (size(s)=w278:i32)
            n106 = local read "Setpoints"() -> (w267:dbl[])
            n107 = Array Size(array=w275) -> (size(s)=w277:i32)
            n108 = Array Subset(array=w276, index=w278, length=w277) -> (w263:dbl[])
            n109 = for {
              N: 4 -> [_]
              tunnel: [w285] -> w265 mode=indexing
              tunnel: w267 -> [w283]
              tunnel: "Subtract Setpoint?" -> [w282]
              tunnel: w263 -> [w280]
              i -> [w284]
              w287 = 7
              n110 = Multiply(x=w287, y=w284) -> (x*y=w286:i32)
              n111 = Index Array(array=w283, index=w284) -> (element=w281:dbl)
              n112 = for {
                N: w287 -> [_]
                tunnel: w286 -> [w294]
                tunnel: w280 -> [w292]
                tunnel: [w288] -> w285 mode=indexing
                tunnel: w282 -> [w291]
                tunnel: w281 -> [w289]
                i -> [w295]
                n113 = Add(x=w294, y=w295) -> (x+y=w293:i32)
                n114 = Index Array(array=w292, index=w293) -> (element=w290:dbl)
                n115 = case shown="False" w291 {
                  tunnel: w290 -> [w296 w299]
                  tunnel: w289 -> [_ w298]
                  tunnel: [w296 w297] -> w288
                  frame False {
                  }
                  frame True {
                    n116 = Subtract(x=w299, y=w298) -> (x-y=w297:dbl)
                  }
                }
              }
            }
            n117 = Array Max & Min(array=w265) -> (min value=w264:dbl)  [unwired: 3 out]
            n118 = call "2D_interpolation.vi"("X Axis Current"=w262, "Min Z Value In"=w264, "Y axis Current"=w261, "Plot In"=w265, "Transpose"=w273, "Point Size"=5) -> ("min Z value"=w271:dbl, "max Z value"=w270:dbl, "Axis info"=w269:T3, "Plot Out"=→"Inlet mapping":dbl[][])  [unwired: 2 in, 4 out]
          }
          frame #1 {
            w305 = u8 0 ("X Scale.Display Format:Precision")
            n119 = Bundle("max Z value"=w309, u32 16721152) -> (w312:cluster{"max Z value":dbl, u32})  [unwired: 1 out]
            n120 = Bundle("min Z value"=w308, u32 3743) -> (w313:cluster{"min Z value":dbl, u32})  [unwired: 1 out]
            n121 = Unbundle By Name(w304) -> ("Y Scale"=w303:cluster{"Xo":dbl, "delta X":dbl}, "Y Max"=w302:dbl, "X Scale"=w301:cluster{"Xo":dbl, "delta X":dbl}, "X Max"=w300:dbl)
            n122 = Build Array(w312, w313) -> (w306:cluster{"min Z value":dbl, u32}[])
            n123 = property on="Inlet mapping" class="IntGraph (strict)"("Ignore Array"=FALSE, "ZScale.MarkerVals[]"=w306, "XScale.Ofst&Mult"=w303, "XScale.Maximum"=w302, "YScale.Ofst&Mult"=w301, "YScale.Maximum"=w300, "XScale.Precision"=w305, "YScale.Precision"=w305) -> ()  [unwired: 2 in, 2 out]
          }
          frame #2 {
            n124 = for {
              N: 5 -> [_]
              tunnel: w320 -> [w328]
              tunnel: w319 -> [w327]
              tunnel: [w322] -> w317 mode=indexing
              i -> [w324]
              w326 = 7 ("length")
              n125 = Multiply(x=w324, y=w326) -> (x*y=w325:i32)
              n126 = Array Subset(array=w327, index=w325, length=w326) -> (w323:dbl[])
              n127 = Bundle("Y Axis Current"=w328, w323) -> (w322:cluster{"Y Axis Current":dbl[], dbl[]})  [unwired: 1 in]
            }
            n128 = local read "Loop number"() -> (w315:i32)
            n129 = Reverse 1D Array(array=w317) -> (reversed array=w316:cluster{"Y Axis Current":dbl[], dbl[]}[])
            n130 = case shown="1, Default" w315 {
              tunnel: w316 -> [_ w321]
              frame 0 {
              }
              frame 1, Default {
                "Lateral profiles" <- w321
              }
            }
          }
        }
        n131 = Build Array (concatenate)(w258, w255) -> (w259:string[])
      }
      frame "EnFlo_Tunnel:Chiller_Pump:Enable" {
        n132 = Array Size(array=w339) -> (size(s)=w337:i32)
        n133 = Index Array(array=w336, index=w337) -> (element=w334:dbl)
        n134 = Greater?(x=w334, y=0.5) -> (0:→"Chiller_Pump:Enable":bool)
        n135 = Build Array (concatenate)(w339, "EnFlo_Tunnel:Chiller_Pump:Enable" ("Ch Name")) -> (w340:string[])
      }
      frame "EnFlo_Tunnel Chilled Water info" {
        n136 = Array Size(array=w366) -> (size(s)=w360:i32)
        n137 = Array Subset(array=w361, index=w360) -> (w359:dbl[])  [unwired: 1 in]
        n138 = Index Array(array=w359) -> (element #1=→"Supply Temp":dbl, element #2=→"Return Temp":dbl, element #3=→"Dem Temp":dbl, element #4=→"Mixing Valve %":dbl, element #5=w346:dbl, element #6=w345:dbl, element #7=→"Heat Exchanger Valve %":dbl, element #8=→"Exit Dem Temp":dbl, element #9=w351:dbl, element #10=w350:dbl, element #11=→"Desired Delta P":dbl, element #12=w343:dbl)  [unwired: 12 in]
        "Supply Pressure" <- w351
        "Return Pressure" <- w350
        n139 = Multiply(x=w343, y=10.0) -> (x*y=→"Pump Speed %":dbl)
        n140 = Max & Min(x=w346, y=w345) -> (max(x,y)=→"Max Motor Temp":dbl)  [unwired: 1 out]
        n141 = Build Array (concatenate)(w366, string[] ["EnFlo_Tunnel:Chilled Water:Supply", "EnFlo_Tunnel:Chilled Water:Return", "EnFlo_Tunnel:Chilled Water:Dem Temp", "EnFlo_Tunnel:Chilled Water:Valve Dem Pos", "EnFlo_Tunnel:Chilled Water:Motor1 Temp", "EnFlo_Tunnel:Chilled Water:Motor2 Temp", "EnFlo_Tunnel:Heat_Ex_Div_Valve:Dem Pos", "EnFlo_Tunnel:Exit Duct:Dem Temp", "EnFlo_Tunnel:Chilled Water:Pressure_supply (Bar)", "EnFlo_Tunnel:Chilled Water:Pressure_return (Bar)", "EnFlo_Tunnel:Chilled Water:Desired_Delta_P", "EnFlo_Tunnel:Chilled Water:Motor_Dem_Voltage"] ("subarray")) -> (w367:string[])
        n142 = Subtract(x=w351, y=w350) -> (x-y=→"Meas Delta P":dbl)
      }
      frame "EnFlo_Tunnel:Floor_Cooling:Enable" {
        n143 = Array Size(array=w379) -> (size(s)=w377:i32)
        n144 = Index Array(array=w376, index=w377) -> (element=w374:dbl)
        n145 = Greater?(x=w374, y=0.5) -> (0:→"Floor_Cooling:Enable":bool)
        n146 = Build Array (concatenate)(w379, "EnFlo_Tunnel:Floor_Cooling:Enable" ("Ch Name")) -> (w380:string[])
      }
      frame "Floor Panels Return Temps" {
        w396 = string[] ["EnFlo_Tunnel:Return_Temp:Floor_Far_02", "EnFlo_Tunnel:Return_Temp:Floor_Near_02", "EnFlo_Tunnel:Return_Temp:Floor_Far_03", "EnFlo_Tunnel:Return_Temp:Floor_Near_03", "EnFlo_Tunnel:Return_Temp:Floor_Far_04", "EnFlo_Tunnel:Return_Temp:Floor_Near_04", "EnFlo_Tunnel:Return_Temp:Floor_Far_05", "EnFlo_Tunnel:Return_Temp:Floor_Near_05", "EnFlo_Tunnel:Return_Temp:Floor_Far_06", "EnFlo_Tunnel:Return_Temp:Floor_Near_06", "EnFlo_Tunnel:Return_Temp:Floor_Far_07", "EnFlo_Tunnel:Return_Temp:Floor_Near_07", "EnFlo_Tunnel:Return_Temp:Floor_Far_08", "EnFlo_Tunnel:Return_Temp:Floor_Near_08", "EnFlo_Tunnel:Return_Temp:Floor_Far_09", "EnFlo_Tunnel:Return_Temp:Floor_Near_09", "EnFlo_Tunnel:Return_Temp:Floor_Far_10", "EnFlo_Tunnel:Return_Temp:Floor_Near_10", "EnFlo_Tunnel:Return_Temp:Floor_Far_11", "EnFlo_Tunnel:Return_Temp:Floor_Near_11", "EnFlo_Tunnel:Return_Temp:Floor_Far_12", "EnFlo_Tunnel:Return_Temp:Floor_Near_12", "EnFlo_Tunnel:Return_Temp:Floor_Far_13", "EnFlo_Tunnel:Return_Temp:Floor_Near_13", "EnFlo_Tunnel:Return_Temp:Floor_Far_14", "EnFlo_Tunnel:Return_Temp:Floor_Turn_14", "EnFlo_Tunnel:Return_Temp:Floor_Turn_Sur_14", "EnFlo_Tunnel:Return_Temp:Floor_Turn_Sur_15", "EnFlo_Tunnel:Return_Temp:Floor_Far_16", "EnFlo_Tunnel:Return_Temp:Floor_Near_16", "EnFlo_Tunnel:Return_Temp:Floor_Far_17", "EnFlo_Tunnel:Return_Temp:Floor_Near_17", "EnFlo_Tunnel:Return_Temp:Floor_Far_18", "EnFlo_Tunnel:Return_Temp:Floor_Near_18", "EnFlo_Tunnel:Return_Temp:Floor_Far_19", "EnFlo_Tunnel:Return_Temp:Floor_Near_19"] ("subarray")
        n147 = Array Size(array=w402) -> (size(s)=w401:i32)
        n148 = local read "Dem Temp"() -> (w390:dbl)
        n149 = for {
          N: 18 -> [_]
          tunnel: [w419] -> w391 mode=indexing
          tunnel: w390 -> [w417]
          tunnel: [w417] -> w389 mode=indexing
          i -> [w420]
          n150 = Add(x=1.5, y=w420) -> (x+y=w419:dbl)
        }
        n151 = Bundle(w391, w389) -> (w385:cluster{dbl[], dbl[]})  [unwired: 1 in]
        n152 = Array Size(array=w396) -> (size(s)=w400:i32)
        n153 = Array Subset(array=w399, index=w401, length=w400) -> (w395:dbl[])
        n154 = Decimate 1D Array(w395) -> (w386:dbl[], w394:dbl[])
        n155 = Not A Number/Path/Refnum?(number/path/refnum=w386) -> (NaN/Path/Refnum?=w388:bool[])
        n156 = And Array Elements(Boolean array=w388) -> (logical AND=w387:bool)
        n157 = Bundle(w391, w386) -> (w393:cluster{dbl[], dbl[]})  [unwired: 1 in]
        n158 = Bundle(w391, w394) -> (w392:cluster{dbl[], dbl[]})  [unwired: 1 in]
        n159 = Build Array(w393, w392, w385) -> (w383:cluster{dbl[], dbl[]}[])
        n160 = case shown="True" w387 {
          tunnel: w385 -> [_ w416]
          tunnel: [w411 w415] -> w384
          tunnel: w383 -> [w411 _]
          frame False {
            n161 = property on="Panel Temps" class="XYGraph (strict)"("Active Plot"=u32 0, "Plot.Plot Name"="Dem Water Temp", "Active Plot"=u32 1, "Plot.Plot Name"="Y-ve Floor Water Return", "Active Plot"=u32 2, "Plot.Plot Name"="Y+ve Floor Water Return") -> ()  [unwired: 2 in, 2 out]
          }
          frame True {
            n162 = property on="Panel Temps" class="XYGraph (strict)"("Active Plot"=u32 0, "Plot.Plot Name"="Dem Water Temp") -> ()  [unwired: 2 in, 2 out]
            n163 = Build Array(w416) -> (w415:cluster{dbl[], dbl[]}[])
          }
        }
        n164 = Build Array (concatenate)(w402, w396) -> (w403:string[])
      }
      frame "Roof Panel Values" {
        w424 = string[] ["EnFlo_Tunnel:Temp:Roof_Far_2", "EnFlo_Tunnel:Temp:Roof_Near_3", "EnFlo_Tunnel:Temp:Roof_Far_4", "EnFlo_Tunnel:Temp:Roof_Far_6", "EnFlo_Tunnel:Temp:Roof_Near_7", "EnFlo_Tunnel:Temp:Roof_Far_8", "EnFlo_Tunnel:Temp:Roof_Far_10", "EnFlo_Tunnel:Temp:Roof_Near_12", "EnFlo_Tunnel:Temp:Roof_Far_15", "EnFlo_Tunnel:Temp:Roof_Far_19"] ("subarray")
        n165 = Array Size(array=w432) -> (size(s)=w431:i32)
        n166 = Array Size(array=w424) -> (size(s)=w430:i32)
        n167 = Array Subset(array=w429, index=w431, length=w430) -> (w425:dbl[])
        n168 = Build Array (concatenate)(w432, w424) -> (w433:string[])
        n169 = Bundle(dbl[] [1.5, 2.5, 3.5, 5.5, 6.5, 7.5, 9.5, 11.5, 14.5, 18.5], w425) -> (w422:cluster{dbl[], dbl[]})  [unwired: 1 in]
        n170 = Build Array (concatenate)(w427, w422) -> (w426:cluster{dbl[], dbl[]}[])
      }
      frame "Upstream Floor Panel Temps" {
        w441 = string[] ["EnFlo_Tunnel:Temp:Floor_Up_Y=-1585", "EnFlo_Tunnel:Temp:Floor_Up_Y=-1250", "EnFlo_Tunnel:Temp:Floor_Up_Y=-920", "EnFlo_Tunnel:Temp:Floor_Up_Y=-585", "EnFlo_Tunnel:Temp:Floor_Up_Y=-250", "EnFlo_Tunnel:Temp:Floor_Up_Y=80", "EnFlo_Tunnel:Temp:Floor_Up_Y=415", "EnFlo_Tunnel:Temp:Floor_Up_Y=750", "EnFlo_Tunnel:Temp:Floor_Up_Y=1080", "EnFlo_Tunnel:Temp:Floor_Up_Y=1415"] ("subarray")
        n171 = Array Size(array=w448) -> (size(s)=w447:i32)
        n172 = Array Size(array=w441) -> (size(s)=w446:i32)
        n173 = Array Subset(array=w445, index=w447, length=w446) -> (w443:dbl[])
        n174 = Build Array (concatenate)(w448, w441) -> (w449:string[])
        n175 = property on="Upstream Floor" class="XYGraph (strict)"("Active Plot"=u32 0, "Plot.Plot Name"="Temp") -> ()  [unwired: 2 in, 2 out]
        n176 = Bundle("Array"=dbl[] [-1585.0, -1250.0, -920.0, -585.0, -250.0, 80.0, 415.0, 750.0, 1080.0, 1415.0], w443) -> (w439:cluster{"Array":dbl[], dbl[]})  [unwired: 1 in]
        n177 = Build Array(w439) -> (w438:cluster{"Array":dbl[], dbl[]}[])
      }
      frame "Upstream Floor Panel Setpoints" {
        w458 = string[] ["EnFlo_Tunnel:Setpoint:Floor_Up_Y=-1585", "EnFlo_Tunnel:Setpoint:Floor_Up_Y=-1250", "EnFlo_Tunnel:Setpoint:Floor_Up_Y=-920", "EnFlo_Tunnel:Setpoint:Floor_Up_Y=-585", "EnFlo_Tunnel:Setpoint:Floor_Up_Y=-250", "EnFlo_Tunnel:Setpoint:Floor_Up_Y=80", "EnFlo_Tunnel:Setpoint:Floor_Up_Y=415", "EnFlo_Tunnel:Setpoint:Floor_Up_Y=750", "EnFlo_Tunnel:Setpoint:Floor_Up_Y=1080", "EnFlo_Tunnel:Setpoint:Floor_Up_Y=1415"] ("subarray")
        n178 = Array Size(array=w465) -> (size(s)=w464:i32)
        n179 = Array Size(array=w454) -> (size(s)=w453:i32)
        n180 = Array Size(array=w458) -> (size(s)=w463:i32)
        n181 = Array Subset(array=w462, index=w464, length=w463) -> (w460:dbl[])
        n182 = Build Array (concatenate)(w465, w458) -> (w466:string[])
        n183 = property on="Upstream Floor" class="XYGraph (strict)"("Active Plot"=w453, "Plot.Plot Name"="Setpoint") -> ()  [unwired: 2 in, 2 out]
        n184 = Bundle("Array"=dbl[] [-1585.0, -1250.0, -920.0, -585.0, -250.0, 80.0, 415.0, 750.0, 1080.0, 1415.0], w460) -> (w456:cluster{"Array":dbl[], dbl[]})  [unwired: 1 in]
        n185 = Build Array (concatenate)(w454, w456) -> (w455:cluster{"Array":dbl[], dbl[]}[])
      }
      frame "Upstream Floor Panel Powers" {
        w475 = string[] ["EnFlo_Tunnel:Power:Floor_Up_Y=-1585", "EnFlo_Tunnel:Power:Floor_Up_Y=-1250", "EnFlo_Tunnel:Power:Floor_Up_Y=-920", "EnFlo_Tunnel:Power:Floor_Up_Y=-585", "EnFlo_Tunnel:Power:Floor_Up_Y=-250", "EnFlo_Tunnel:Power:Floor_Up_Y=80", "EnFlo_Tunnel:Power:Floor_Up_Y=415", "EnFlo_Tunnel:Power:Floor_Up_Y=750", "EnFlo_Tunnel:Power:Floor_Up_Y=1080", "EnFlo_Tunnel:Power:Floor_Up_Y=1415"] ("subarray")
        n186 = Array Size(array=w482) -> (size(s)=w481:i32)
        n187 = Array Size(array=w471) -> (size(s)=w470:i32)
        n188 = Array Size(array=w475) -> (size(s)=w480:i32)
        n189 = Array Subset(array=w479, index=w481, length=w480) -> (w477:dbl[])
        n190 = Build Array (concatenate)(w482, w475) -> (w483:string[])
        n191 = property on="Upstream Floor" class="XYGraph (strict)"("Active Plot"=w470, "Plot.Plot Name"="Power") -> ()  [unwired: 2 in, 2 out]
        n192 = Bundle("Array"=dbl[] [-1585.0, -1250.0, -920.0, -585.0, -250.0, 80.0, 415.0, 750.0, 1080.0, 1415.0], w477) -> (w473:cluster{"Array":dbl[], dbl[]})  [unwired: 1 in]
        n193 = Build Array (concatenate)(w471, w473) -> (w472:cluster{"Array":dbl[], dbl[]}[])
      }
      frame "Upstream Above Floor Panel" {
        w492 = string[] ["EnFlo_Tunnel:Temp:Z=70_Y=-1585", "EnFlo_Tunnel:Temp:Z=70_Y=-1250", "EnFlo_Tunnel:Temp:Z=70_Y=-920", "EnFlo_Tunnel:Temp:Z=70_Y=-585", "EnFlo_Tunnel:Temp:Z=70_Y=-250", "EnFlo_Tunnel:Temp:Z=70_Y=80", "EnFlo_Tunnel:Temp:Z=70_Y=415", "EnFlo_Tunnel:Temp:Z=70_Y=750", "EnFlo_Tunnel:Temp:Z=70_Y=1080", "EnFlo_Tunnel:Temp:Z=70_Y=1415"] ("subarray")
        n194 = Array Size(array=w499) -> (size(s)=w498:i32)
        n195 = Array Size(array=w488) -> (size(s)=w487:i32)
        n196 = Array Size(array=w492) -> (size(s)=w497:i32)
        n197 = Array Subset(array=w496, index=w498, length=w497) -> (w494:dbl[])
        n198 = Build Array (concatenate)(w499, w492) -> (w500:string[])
        n199 = property on="Upstream Floor" class="XYGraph (strict)"("Active Plot"=w487, "Plot.Plot Name"="Z=70") -> ()  [unwired: 2 in, 2 out]
        n200 = Bundle("Array"=dbl[] [-1585.0, -1250.0, -920.0, -585.0, -250.0, 80.0, 415.0, 750.0, 1080.0, 1415.0], w494) -> (w490:cluster{"Array":dbl[], dbl[]})  [unwired: 1 in]
        n201 = Build Array (concatenate)(w488, w490) -> (w489:cluster{"Array":dbl[], dbl[]}[])
      }
      frame "Lab Stratification" {
        w519 = dbl[] [0.0, 6.0]
        w522 = 8 ("length")
        w534 = dbl[] [5.75, 4.5, 3.5, 2.5, 1.5, 0.5, 0.1, 0.0]
        n202 = Array Size(array=w537) -> (size(s)=w521:i32)
        n203 = Add(x=w521, y=w522) -> (x+y=w520:i32)
        n204 = Array Subset(array=w524, index=w520) -> (w523:dbl[])  [unwired: 1 in]
        n205 = Index Array(array=w523) -> (element #1=→"Delta T":dbl, element #2=w516:dbl, element #3=→"Heat Extraction kW":dbl, element #4=w518:dbl)  [unwired: 4 in]
        "Av Pre Inlet Temp" <- w516
        "Des Air Temp" <- w518
        n206 = Array Subset(array=w524, index=w521, length=w522) -> (w527:dbl[])
        n207 = for {
          N: 15 -> [_]
          tunnel: 2.43 -> [w545]
          tunnel: [w543] -> w531 mode=indexing
          i -> [w547]
          n208 = Multiply(x=0.1, y=w547) -> (x*y=w544:dbl)
          n209 = Subtract(x=w545, y=w544) -> (x-y=w543:dbl)
        }
        n210 = call <vilib>:"Interpolate 1D.vi"("xi"=w531, "X"=w534, "Y"=w527) -> ("yi"=w530:dbl[])  [unwired: 3 in, 5 out]
        n211 = Build Array(w518, w518) -> (w517:dbl[])
        n212 = Build Array(w516, w516) -> (w515:dbl[])
        n213 = local read "Heaters Enabled"() -> (w506:bool)
        n214 = Bundle(w527, w534) -> (w514:cluster{dbl[], dbl[]})  [unwired: 1 in]
        n215 = Bundle(w517, w519) -> (w513:cluster{dbl[], dbl[]})  [unwired: 1 in]
        n216 = Bundle(w515, w519) -> (w512:cluster{dbl[], dbl[]})  [unwired: 1 in]
        n217 = Bundle("yi"=w530, w510) -> (w529:cluster{"yi":dbl[], dbl[]})  [unwired: 1 in]
        n218 = case shown="False" w506 {
          tunnel: ["Get Server Values" "Inlet Heater Setpoint Values"] -> w505
          frame False {
          }
          frame True {
          }
        }
        n219 = Build Array(w514, w513, w512) -> (w511:cluster{dbl[], dbl[]}[])
        n220 = Build Array (concatenate)(w537, string[] ["EnFlo Lab:labstrat1:Z=5.75m Roof", "EnFlo Lab:labstrat1:Z=4.5m", "EnFlo Lab:labstrat1:Z=3.5m", "EnFlo Lab:labstrat1:Z=2.5m", "EnFlo Lab:labstrat1:Z=1.5m", "EnFlo Lab:labstrat1:Z=0.5m", "EnFlo Lab:labstrat1:Z=0.1m", "EnFlo Lab:labstrat1:Z=0m Floor", "EnFlo Lab:labstrat1:Delta T", "EnFlo_Tunnel:Temp:Pre_Inlet_Average", "EnFlo Lab:Heat:Extraction", "EnFlo Lab:Desired:Air Temp"] ("subarray")) -> (w538:string[])
        n221 = local read "Loop number"() -> (w504:i32)
        n222 = case shown="1, Default" w504 {
          tunnel: w511 -> [_ w540]
          frame 0 {
          }
          frame 1, Default {
            "Strat" <- w540
          }
        }
        n223 = Array Size(array=w507) -> (size(s)=w508:i32)
        n224 = Build Array (concatenate)(w507, w529) -> (w528:cluster{"yi":dbl[], dbl[]}[])
        n225 = property on="Inlet Heaters" class="XYGraph (strict)"("Active Plot"=w508, "Plot.Plot Name"="Lab Strat") -> ()  [unwired: 2 in, 2 out]
      }
      frame "Inlet Heater Setpoint Values" {
        w549 = string[] ["EnFlo_Tunnel:Setpoint:Inlet_Y=0_Z=1450", "EnFlo_Tunnel:Setpoint:Inlet_Y=0_Z=1350", "EnFlo_Tunnel:Setpoint:Inlet_Y=0_Z=1250", "EnFlo_Tunnel:Setpoint:Inlet_Y=0_Z=1150", "EnFlo_Tunnel:Setpoint:Inlet_Y=0_Z=1050", "EnFlo_Tunnel:Setpoint:Inlet_Y=0_Z=950", "EnFlo_Tunnel:Setpoint:Inlet_Y=0_Z=850", "EnFlo_Tunnel:Setpoint:Inlet_Y=0_Z=750", "EnFlo_Tunnel:Setpoint:Inlet_Y=0_Z=650", "EnFlo_Tunnel:Setpoint:Inlet_Y=0_Z=550", "EnFlo_Tunnel:Setpoint:Inlet_Y=0_Z=450", "EnFlo_Tunnel:Setpoint:Inlet_Y=0_Z=350", "EnFlo_Tunnel:Setpoint:Inlet_Y=0_Z=250", "EnFlo_Tunnel:Setpoint:Inlet_Y=0_Z=150", "EnFlo_Tunnel:Setpoint:Inlet_Y=0_Z=50"] ("subarray")
        n226 = Array Size(array=w564) -> (size(s)=w563:i32)
        n227 = Array Size(array=w552) -> (size(s)=w550:i32)
        n228 = property on="Inlet Heaters" class="XYGraph (strict)"("Active Plot"=w550, "Plot.Plot Name"="Inlet Setpoints") -> ()  [unwired: 2 in, 2 out]
        n229 = Array Size(array=w549) -> (size(s)=w562:i32)
        n230 = Array Subset(array=w561, index=w563, length=w562) -> (w554:dbl[])
        n231 = Bundle(w554, w553) -> (w560:cluster{dbl[], dbl[]})  [unwired: 1 in]
        n232 = for {
          tunnel: i32[] [14, 10, 5, 0] -> [w569] mode=indexing
          tunnel: w554 -> [w567]
          tunnel: [w568] -> w556 mode=indexing
          n233 = Index Array(array=w567, index=w569) -> (element=w568:dbl)
        }
        "Setpoints" <- w556
        n234 = Build Array (concatenate)(w564, w549) -> (w565:string[])
        n235 = Build Array (concatenate)(w552, w560) -> (w559:cluster{"yi":dbl[], dbl[]}[])
      }
      frame "Inlet Heater Power Values" {
        w571 = string[] ["EnFlo_Tunnel:Power:Inlet_Y=0_Z=1450", "EnFlo_Tunnel:Power:Inlet_Y=0_Z=1350", "EnFlo_Tunnel:Power:Inlet_Y=0_Z=1250", "EnFlo_Tunnel:Power:Inlet_Y=0_Z=1150", "EnFlo_Tunnel:Power:Inlet_Y=0_Z=1050", "EnFlo_Tunnel:Power:Inlet_Y=0_Z=950", "EnFlo_Tunnel:Power:Inlet_Y=0_Z=850", "EnFlo_Tunnel:Power:Inlet_Y=0_Z=750", "EnFlo_Tunnel:Power:Inlet_Y=0_Z=650", "EnFlo_Tunnel:Power:Inlet_Y=0_Z=550", "EnFlo_Tunnel:Power:Inlet_Y=0_Z=450", "EnFlo_Tunnel:Power:Inlet_Y=0_Z=350", "EnFlo_Tunnel:Power:Inlet_Y=0_Z=250", "EnFlo_Tunnel:Power:Inlet_Y=0_Z=150", "EnFlo_Tunnel:Power:Inlet_Y=0_Z=50"] ("subarray")
        n236 = Array Size(array=w584) -> (size(s)=w583:i32)
        n237 = Array Size(array=w573) -> (size(s)=w574:i32)
        n238 = Array Size(array=w571) -> (size(s)=w582:i32)
        n239 = Array Subset(array=w581, index=w583, length=w582) -> (w580:dbl[])
        n240 = Bundle(w580, w578) -> (w576:cluster{dbl[], dbl[]})  [unwired: 1 in]
        n241 = Build Array (concatenate)(w584, w571) -> (w585:string[])
        n242 = property on="Inlet Heaters" class="XYGraph (strict)"("Active Plot"=w574, "Plot.Plot Name"="Inlet Powers") -> ()  [unwired: 2 in, 2 out]
        n243 = Build Array (concatenate)(w573, w576) -> (w577:cluster{"yi":dbl[], dbl[]}[])
      }
      frame "Get Server Values" {
        n244 = local read "Loop number"() -> (w588:i32)
        n245 = Increment(x=w588) -> (x+1=w592:i32)
        n246 = local write "Loop number"(w592) -> ()
        n247 = case shown="Default" w588 {
          tunnel: w591 -> [_ w606 _]
          tunnel: [TRUE ("Top Level") w604 w639] -> w594
          frame 0 {
          }
          frame 1 {
            n248 = global read "Constants_global.vi" "Data Folder Local"() -> (w605:path)
            n249 = stacked-sequence {
              tunnel: w606 -> [w615 _]
              tunnel: w605 -> [w609 w632]
              tunnel: [w607 _] -> w604
              frame #0 {
                n250 = for {
                  tunnel: T2 {"Template Channel Name"="", "Description"="", "Tolerance"=0.0, "Precision"="", "Folder level"="", "Source"=[], "Replace"=[], "Summarise"=FALSE, "Dispose"=FALSE, "Minimum Value"="", "Maths"="", "Omit Rows Containing"=[], "Ignore When"=[]} ("Cluster") -> [w625]
                  tunnel: w615 -> [w618] mode=indexing
                  tunnel: [w624] -> w614 mode=indexing if=w620
                  shift-right: [w622] -> _
                  shift-left: string[] [] -> [w623]
                  tunnel: "Do not prompt me if this channnel is not found" -> [w617]
                  n251 = Search 1D Array(1D array=w623, element=w618) -> (index of element=w621:i32)  [unwired: 1 in]
                  n252 = Build Array(w618, w617) -> (w619:string[])
                  n253 = Bundle By Name(cluster=w625, "Template Channel Name"=w618, "Source"=w619) -> (w624:T2)
                  n254 = case shown="-1" w621 {
                    tunnel: w623 -> [w627 w631]
                    tunnel: [w627 w630] -> w622
                    tunnel: w618 -> [_ w629]
                    tunnel: [FALSE TRUE] -> w620
                    frame Default {
                    }
                    frame -1 {
                      n255 = Build Array (concatenate)(w631, w629) -> (w630:string[])
                    }
                  }
                }
                n256 = Build Path(base path=w609, name or relative path="EnFlo_Tunnel_Display_Template.xls") -> (appended path=w610:path)
                n257 = local read "Top Level"() -> (w607:bool)
                n258 = call "Read_Write_Temp_Cluster.vi"("Template Info Array"=w614, "Mode"=Global_mode."Write Global to File", "Template File"=w610) -> ()  [unwired: 2 in, 1 out]
              }
              frame #1 {
                n259 = Path To String(path=w632) -> (string=w633:string)
                n260 = call "Read_Write_Template.vi"("Mode"=Global_mode."Write Global to File", "Single Value In"=w633, "Data type"="Log Folder Name" ("Variable name")) -> ()  [unwired: 5 in, 8 out]
              }
            }
          }
          frame Default {
            n261 = global read "Results_plotter_Global.vi" "Plot EnFlo Tunnel Display"() -> (w638:bool)
            n262 = Or(x=w638, y="Stop Button") -> (x .or. y?=w636:bool)
            n263 = Not(x=w636) -> (.not. x?=w639:bool)
          }
        }
        n264 = Multiply(x="History in Minutes", y=60.0) -> (x*y=w597:dbl)
        n265 = call "Get_Channel_averages.vi"("Desired Ch Names"=w591, "Averaging time (mins)"="Averaging time (mins)", "End Offset Sec (0)"=w597) -> ("number"=w593:dbl[])  [unwired: 2 out]
        n266 = case shown="1, Default" w588 {
          tunnel: w590 -> [_ w602]
          tunnel: w589 -> [_ w601]
          tunnel: w587 -> [_ w600]
          frame 0 {
          }
          frame 1, Default {
            "Inlet Heaters" <- w601
            "Panel Temps" <- w602
            "Upstream Floor" <- w600
          }
        }
      }
    }
  }
